vi "ProdaNG.Configurator.vi"() -> ()   [LabVIEW 2016]
uses:
  ProdaNG.Tree.TestViewMode.ctl
  ProdaNG.File.Sequence.ctl
  ProdaNG.Tree.Fglb.Value.ctl
  ProdaNG.File.Step.ctl
  ProdaNG.Configurator.DB.ctl
  ProdaNG.Configurator.Config.ctl
  ProdaNG.Configurator.ResultsTimeSpan.ctl
  Controls/ProdaNG.Product.ctl
  ProdaNG.Configurator.State.ctl
  <vilib>/Utility/error.llb/DialogTypeEnum.ctl
  <vilib>/Utility/miscctls.llb/LVNodeAndColumnTypeDef.ctl
  ProdaNG.Configurator.Glb.vi
panel:
  out "Products":T1[](array[typedef])
  out "DBtime":timestamp
  out "SelectedFile":path
  out "Progress":bool caption="Please wait..."
  out "Hider":bool
  out "PrevTabState":i32
  in  "ButtonResults":bool
  out "SlotInUse":i32
  in  "ButtonTest":bool
  in  "ButtonParts":bool
  out "DB":T2
  out "ProfInfo":string[](array[string])
  in  "TestTreeView":T3
  out "FPref":refnum<vi>
  out "FileContent":T4
  in  "MainTab":enum32{"Parts", "Test", "Results"}(tab)
  in  "ButtonConnect":bool caption="Check"
  out "HiderParts":bool
  in  "ButtonGoToResults":bool
  in  "ButtonGoToTest":bool caption="Accept"
  in  "VariantFilter":string caption="Wabco Part Filter"
  in  "ButtonRefreshTreeProc":bool caption="Refresh"
  in  "ProcTree":string(tree) caption="Found 4 wabco parts"
  out "Identification":T7
  out "Process Found":bool
  in  "color legend 4":u32(colorbox)=16448250 caption="- wabco part"
  in  "color legend 5":u32(colorbox)=12058551 caption="- process"
  in  "color legend 6":u32(colorbox)=16777134 caption="- process step"
  in  "ButtonReloadDB":bool caption="Refresh"
  in  "Configuration":T8={"ShowUnreleased"=TRUE, "Param1"="StepIndex", "ParamStartIdx"=0, "Slots"=1} {"Slots" min=1 max=2; "ParamStartIdx" min=0 max=1}
  in  "TestTree.OpenCloseAll":bool caption="collapse all"
  in  "ButtonSaveToFile":bool
  out "FileInUse":string
  in  "ButtonCloseFile":bool
  in  "ButtonExportFile":bool
  in  "ButtonOpenFile":bool
  in  "color legend 1":u32(colorbox)=16448250 caption="- item synchronized"
  in  "color legend 3":u32(colorbox)=16744576 caption="- item value changed"
  in  "color legend 2":u32(colorbox)=16777147 caption="- new item in file (not found in DB)"
  in  "ButtonUnreleaseAll":bool
  in  "ButtonReleaseAll":bool
  in  "ButtonUnrelease":bool
  in  "ButtonRelease":bool
  in  "ButtonDeleteAll":bool
  in  "ButtonAdd":bool
  in  "ButtonEdit":bool
  in  "ButtonDelete":bool
  in  "TestTree":string[](tree)
  in  "ButtonRefreshTestTree":bool
  in  "ResultsAmount":i32 caption="Span" min=0 max=100
  in  "ResultsSpan":T9
  in  "Results.TimeTo":timestamp caption="Time To" format="%<%x %X>T"
  in  "Results.TimeFrom":timestamp caption="Time From" format="%<%x %X>T"
  in  "ProductList":i32[](listbox) caption="Products #208"
  in  "color legend 9":u32(colorbox)=16448250 caption="- value ok"
  in  "color legend 8":u32(colorbox)=16744576 caption="- value nok"
  in  "color legend 7":u32(colorbox)=13816530 caption="- value missing"
  in  "ResultsTree":string[](tree)
  in  "ButtonRefreshResultTree":bool
  in  "ProductListSelectAll":enum8{"False", "True", "Mixed"}(c332) caption="All"
  in  "Starthere":bool
  out "Status":string
  out "DBStatus":string
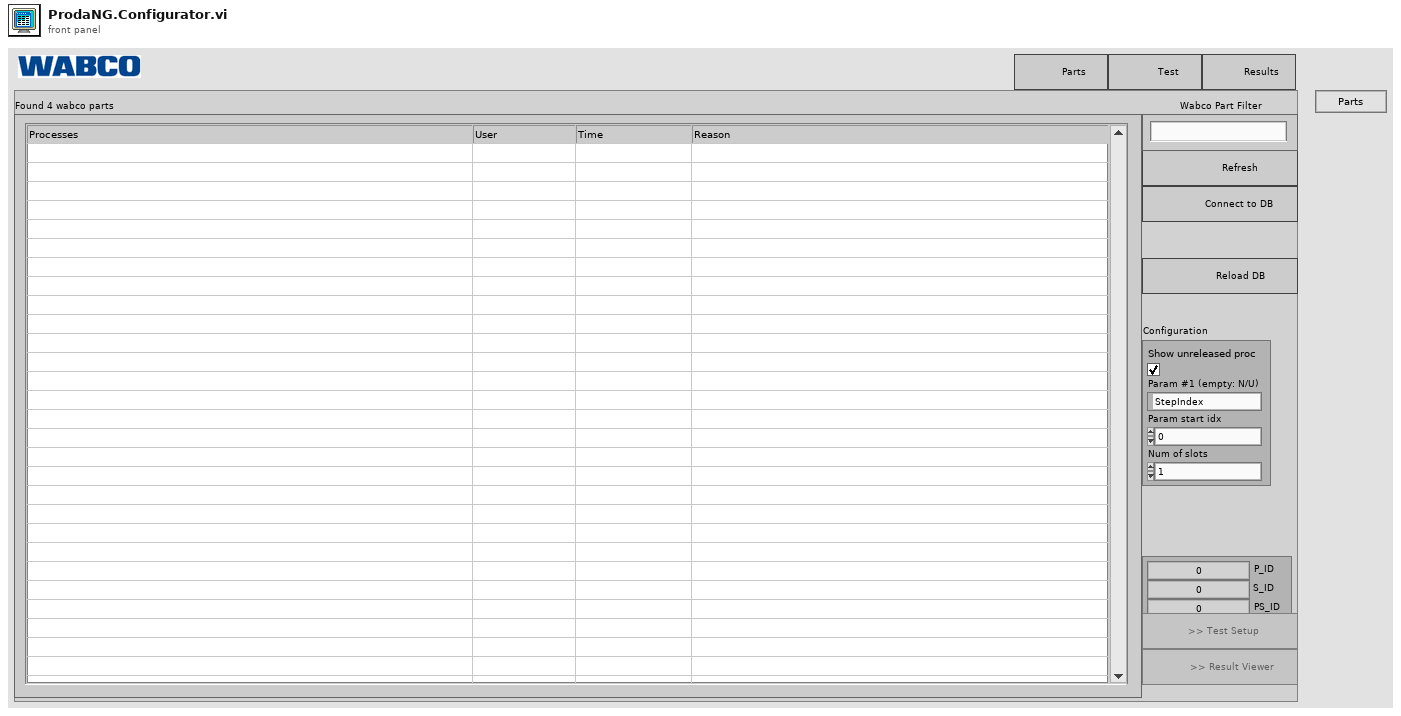
[diagram p1: front panel]
types:
  T1 = typedef "ProdaNG.Product.ctl" = cluster{"c_id":string, "wabcoPartId":i32, "serialNumber":string, "comment":string, "individual":i32, "crProcessStepId":i32, "mdProcessStepId":i32, "crTime":string, "mdTime":string}
  T2 = typedef "ProdaNG.Configurator.DB.ctl" = enum16{"other", "WPL", "WPK"}
  T3 = typedef "ProdaNG.Tree.TestViewMode.ctl" = enum16{"All", "Released", "Unreleased"}
  T4 = typedef "ProdaNG.File.Sequence.ctl" = cluster{"PP":T5[], "TS":T6[]}
  T5 = typedef "ProdaNG.Tree.Fglb.Value.ctl" = cluster{"desc":string, "order":i32, "value1":dbl, "value2":dbl, "unit":i32}
  T6 = typedef "ProdaNG.File.Step.ctl" = cluster{"TS":T5, "TP":T5[], "TV":T5[]}
  T7 = cluster{"P_ID":i32, "S_ID":i32, "PS_ID":i32, "WP_ID":i32}
  T8 = typedef "ProdaNG.Configurator.Config.ctl" = cluster{"ShowUnreleased":bool, "Param1":string, "ParamStartIdx":i32, "Slots":i32}
  T9 = typedef "ProdaNG.Configurator.ResultsTimeSpan.ctl" = enum16{"Custom", "Shift(s)", "Hour(s)", "Day(s)", "Week(s)", "Month(s)"}
  T10 = typedef "ProdaNG.Configurator.State.ctl" = enum16{"Disconnected", "Connected", "ProcessFound"}
  T11 = enum8{"Enabled", "Disabled", "Disabled and Grayed Out"}
  T12 = cluster{"processId":i32, "systemId":i32, "processStepId":i32, "wabcoPartId":i32}
  T13 = typedef "DialogTypeEnum.ctl" = enum16{"no dialog", "OK message", "continue or stop message", "auto error handling dialog", "OK message + warnings", "continue/stop + warnings"}
  T14 = typedef "LVNodeAndColumnTypeDef.ctl" = cluster{"Node":string, "Column":i32}
  T15 = enum16{"Custom", "Shift(s)", "Hour(s)", "Day(s)", "Week(s)", "Month(s)"}
  T16 = typedef "LVPositionTypeDef.ctl" = cluster{"Left":i32, "Top":i32}
  T17 = typedef "ProdaNG.ProdutionLine.ctl" = cluster{"i_id":i32, "description":string}
  T18 = typedef "ProdaNG.System.ctl" = cluster{"i_id":i32, "description":string}
  T19 = typedef "ProdaNG.Process.ctl" = cluster{"i_id":i32, "productionLineId":i32, "releaseId":i32, "contentId":string, "previewId":string, "mdReason":string, "mdUser":string, "mdTime":string, "description":string}
  T20 = typedef "ProdaNG.WabcoPart.ctl" = cluster{"i_id":i32, "workCenterId":i32, "contentId":string, "previewId":string, "mdReason":string, "mdUser":string, "mdTime":string, "productName":string, "wabcoNumber":string}
  T21 = typedef "ProdaNG.ProcessStep.ctl" = cluster{"i_id":i32, "processId":i32, "systemId":i32, "releaseId":i32, "processSequence":i32, "limitYellow":dbl, "limitRed":dbl, "mdReason":string, "mdUser":string, "mdTime":string, "filename":string, "transfer":string, "description":string}
  T22 = typedef "ProdaNG.Tree.Fglb.Data.ctl" = cluster{"tag":string, "row":i32, "element":T23, "idx1":i32, "idx2":i32, "file":bool}
  T23 = typedef "ProdaNG.Tree.Fglb.Element.ctl" = enum16{"-", "PP", "TS", "TP", "TV"}
  T24 = typedef "ProdaNG.UnitSimple.ctl" = cluster{"name":string, "i_id":i32}
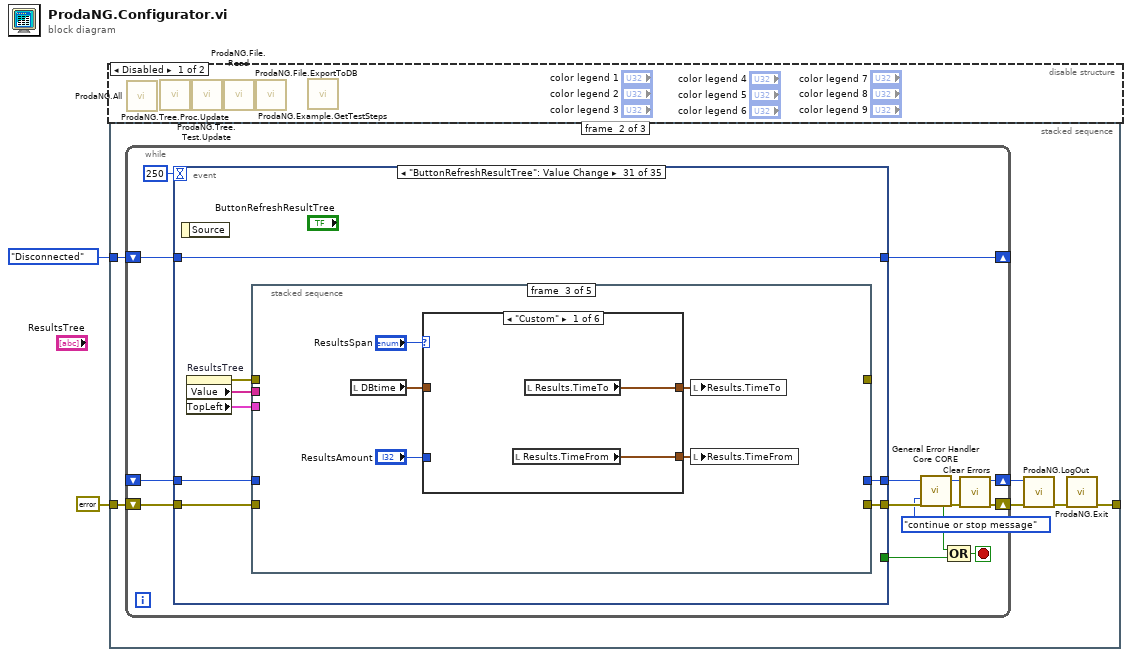
[diagram p0: block diagram]
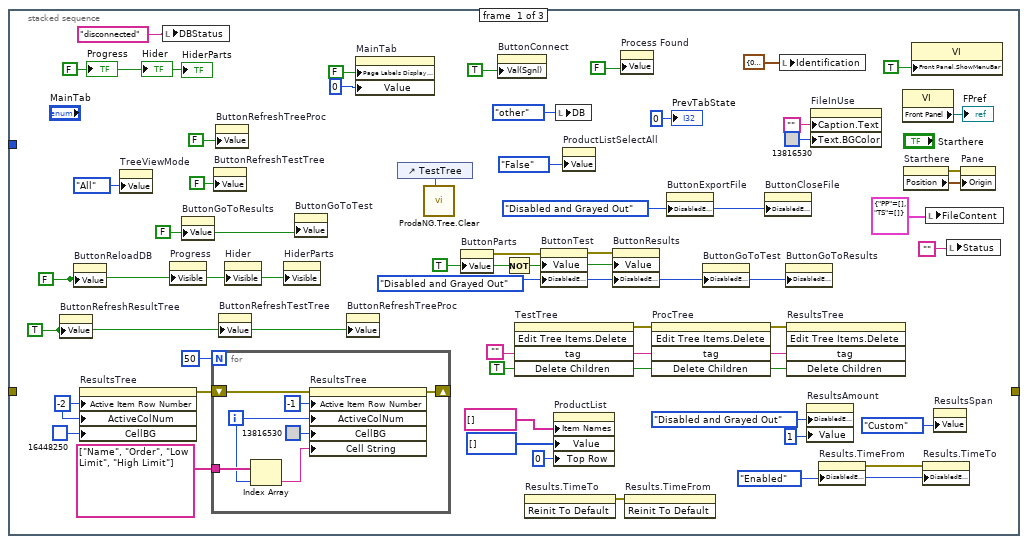
[diagram p2: hidden frame]
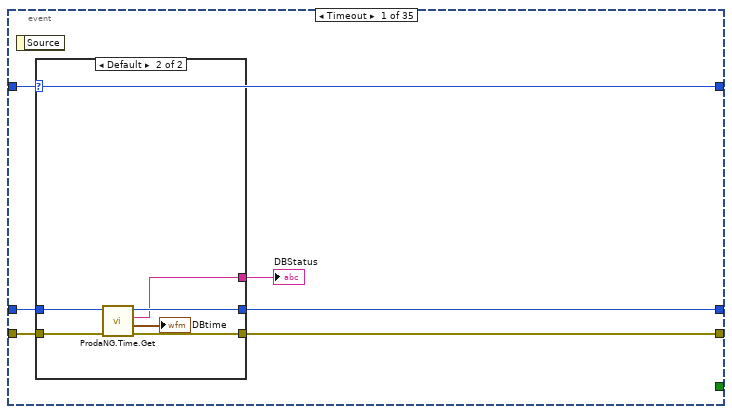
[diagram p3: hidden frame]
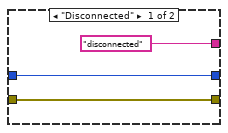
[diagram p4: hidden frame]
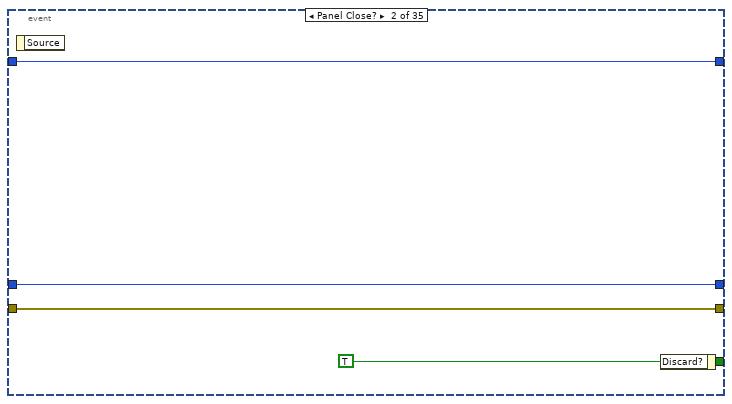
[diagram p5: hidden frame]
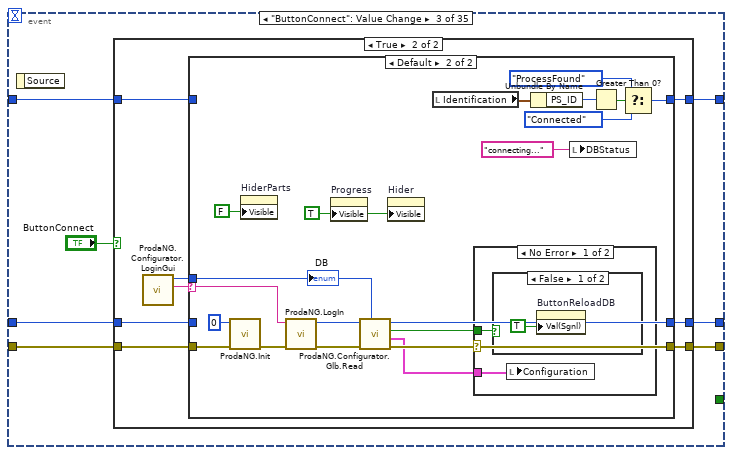
[diagram p6: hidden frame]
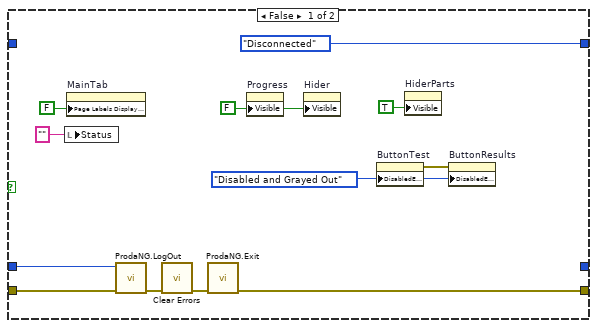
[diagram p7: hidden frame]
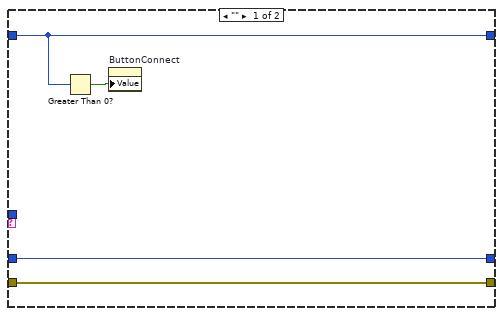
[diagram p8: hidden frame]
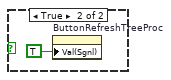
[diagram p9: hidden frame]
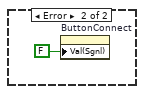
[diagram p10: hidden frame]
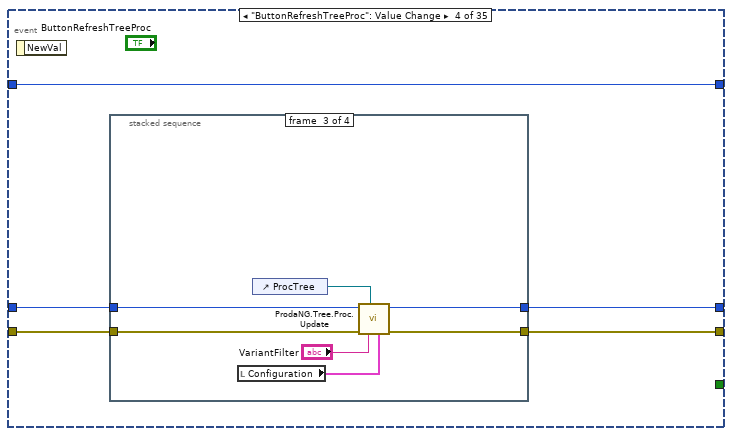
[diagram p11: hidden frame]
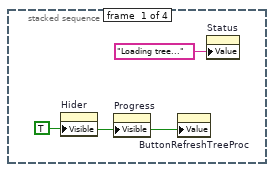
[diagram p12: hidden frame]
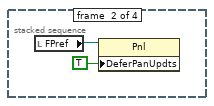
[diagram p13: hidden frame]
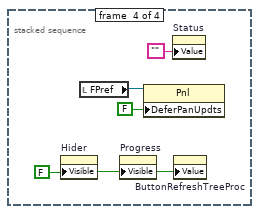
[diagram p14: hidden frame]
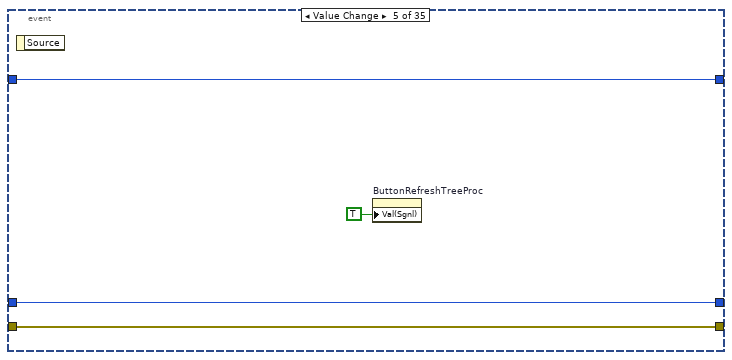
[diagram p15: hidden frame]
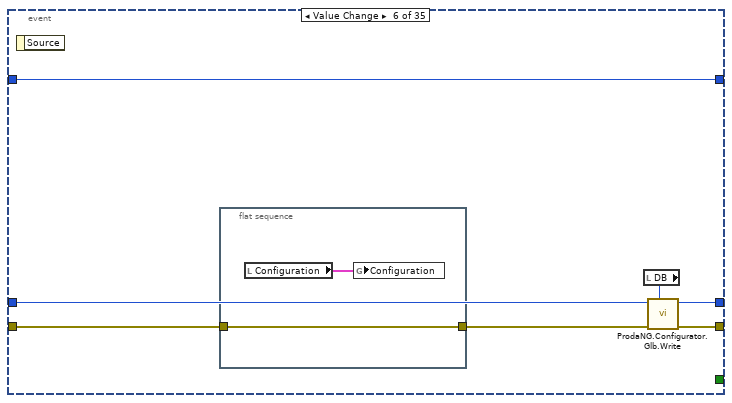
[diagram p16: hidden frame]
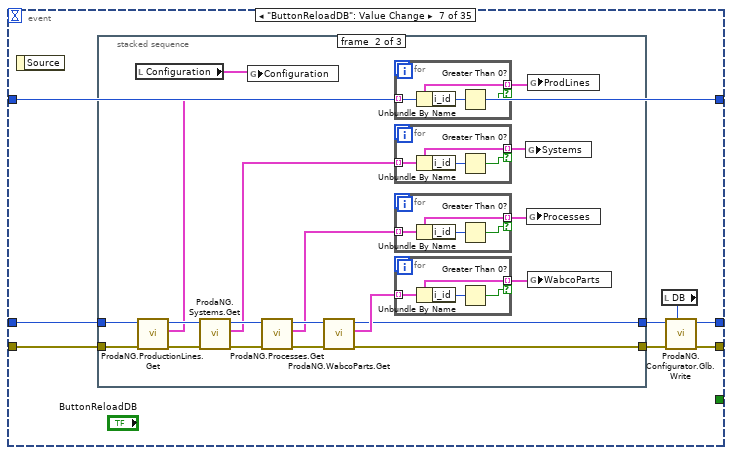
[diagram p17: hidden frame]
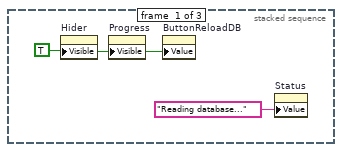
[diagram p18: hidden frame]
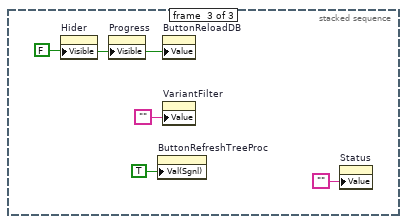
[diagram p19: hidden frame]
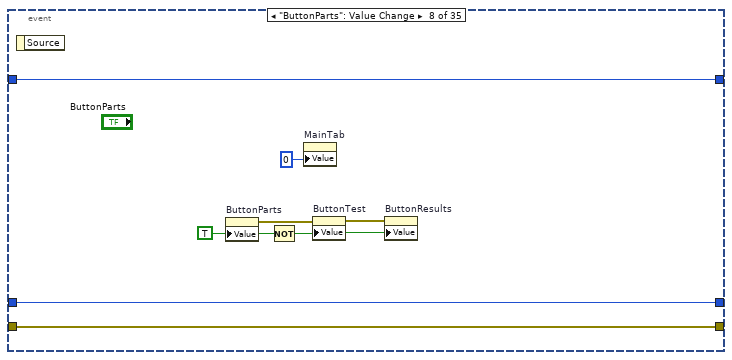
[diagram p20: hidden frame]
diagram:
  n1 = disable-structure shown="Disabled" {
    frame Disabled {
      n2 = call "ProdaNG.All.vi"() -> ()  [unwired: 1 in]
      n3 = call "ProdaNG.Tree.Proc.Update.vi"() -> ()  [unwired: 10 in, 2 out]
      n4 = call "ProdaNG.Tree.Test.Update.vi"() -> ()  [unwired: 8 in, 4 out]
      n5 = call "ProdaNG.File.Read.vi"() -> ()  [unwired: 9 in, 3 out]
      n6 = call "ProdaNG.File.ExportToDB.vi"() -> ()  [unwired: 10 in, 2 out]
      n7 = call "ProdaNG.Example.GetTestSteps.vi"() -> ()  [unwired: 12 in]
    }
    frame Enabled {
    }
  }
  n8 = stacked-sequence {
    tunnel: ProdaNG.Configurator.State."Disconnected" ("State") -> [_ w62 _]
    tunnel: [_ w60 _] -> _
    tunnel: errorcluster {"status"=FALSE, "code"=0, "source"=""} ("error out") -> [_ w59 _]
    frame #0 {
      w5 = T11."Enabled" ("Disabled")
      w11 = TRUE ("Value (Signaling)")
      w17 = -2 ("Active Item:Row Number")
      w23 = TRUE ("Delete Children?")
      w24 = ""
      w28 = FALSE ("Progress")
      w29 = FALSE ("ButtonGoToResults")
      w31 = T11."Disabled and Grayed Out" ("Disabled")
      w36 = TRUE ("ButtonPartList")
      w27 = FALSE ("Visible")
      w45 = T11."Disabled and Grayed Out" ("Disabled")
      n9 = property on="ButtonRefreshResultTree" class="Bool (strict)"("Value"=w11) -> ()  [unwired: 2 in, 2 out]
      n10 = property on="ButtonReloadDB" class="Bool (strict)"("Value"=w27) -> ()  [unwired: 2 in, 2 out]
      n11 = property on="ResultsTree" class="Tree (strict)"("Active Item Row Number"=w17, "ActiveColNum"=w17, "CellBG"=u32 16448250) -> (error out=w18:errorcluster)  [unwired: 2 in, 1 out]
      n12 = property on="TreeViewMode" class="Enum (strict)"("Value"=ProdaNG.Tree.TestViewMode."All" ("TreeViewMode")) -> ()  [unwired: 2 in, 2 out]
      n13 = local write "DBStatus"("disconnected" ("string")) -> ()
      n14 = property on="Progress" class="Bool (strict)"("Visible"=w27) -> ()  [unwired: 2 in, 2 out]
      n15 = property on="ButtonGoToResults" class="Bool (strict)"("Value"=w29) -> ()  [unwired: 2 in, 2 out]
      n16 = for {
        N: 50 -> [_]
        tunnel: string[] ["Name", "Order", "Low Limit", "High Limit"] -> [w55]
        shift-right: [w53] -> _
        shift-left: w18 -> [w58]
        i -> [w52]
        n17 = Index Array(array=w55, index=w52) -> (element=w54:string)
        n18 = property on="ResultsTree" class="Tree (strict)"(error in=w58, "Active Item Row Number"=-1 ("Active Item:Row Number"), "ActiveColNum"=w52, "CellBG"=u32 13816530, "Cell String"=w54) -> (error out=w53:errorcluster)  [unwired: 1 in, 1 out]
      }
      n19 = property on="ButtonRefreshTestTree" class="Bool (strict)"("Value"=FALSE ("ButtonRefreshSystem")) -> ()  [unwired: 2 in, 2 out]
      n20 = property on="ButtonRefreshTreeProc" class="Bool (strict)"("Value"=FALSE ("Value (Signaling)")) -> ()  [unwired: 2 in, 2 out]
      n21 = property on="ButtonRefreshTestTree" class="Bool (strict)"("Value"=w11) -> ()  [unwired: 2 in, 2 out]
      n22 = property on="Hider" class="Bool (strict)"("Visible"=w27) -> ()  [unwired: 2 in, 2 out]
      n23 = property on="HiderParts" class="Bool (strict)"("Visible"=w27) -> ()  [unwired: 2 in, 2 out]
      n24 = property on="ButtonGoToTest" class="Bool (strict)"("Value"=w29) -> ()  [unwired: 2 in, 2 out]
      n25 = property on="ButtonRefreshTreeProc" class="Bool (strict)"("Value"=w11) -> ()  [unwired: 2 in, 2 out]
      n26 = property on="MainTab" class="TabCtl (strict)"("Page Labels Display Visible?"=FALSE, "Value"=0) -> ()  [unwired: 2 in, 2 out]
      n27 = control-ref of="TestTree"() -> (w49:refnum<vi>)
      n28 = call "ProdaNG.Tree.Clear.vi"("TestStepsTree"=w49) -> ()  [unwired: 10 in, 1 out]
      n29 = property on="ButtonParts" class="Bool (strict)"("Value"=w36) -> (error out=w35:errorcluster)  [unwired: 2 in, 1 out]
      n30 = property on="ButtonConnect" class="Bool (strict)"("Val(Sgnl)"=TRUE ("ButtonConnect")) -> ()  [unwired: 2 in, 2 out]
      n31 = Not(x=w36) -> (.not. x?=w33:bool)
      n32 = invoke on="TestTree" class="Tree (strict)" method="Edit Tree Items.Delete"("tag"=w24, "Delete Children"=w23) -> (error out=w26:errorcluster)  [unwired: 3 in, 4 out]
      n33 = invoke on="Results.TimeTo" class="AbsTime (strict)" method="Reinit To Default"() -> (error out=w3:errorcluster)  [unwired: 3 in, 2 out]
      n34 = property on="ButtonTest" class="Bool (strict)"(error in=w35, "Value"=w33, "DisabledEnum"=w31) -> (error out=w34:errorcluster)  [unwired: 1 in, 1 out]
      n35 = property on="ProductList" class="LstBox (strict)"("Item Names"=string[] [], "Value"=i32[] [] ("ProductList"), "Top Row"=0) -> ()  [unwired: 2 in, 2 out]
      n36 = local write "DB"(ProdaNG.Configurator.DB."other" ("DB")) -> ()
      n37 = property on="ProductListSelectAll" class="MixedCheckbox (strict)"("Value"=enum8{"False", "True", "Mixed"}."False" ("Mixed Checkbox")) -> ()  [unwired: 2 in, 2 out]
      n38 = property on="ButtonResults" class="Bool (strict)"(error in=w34, "Value"=w33, "DisabledEnum"=w31) -> ()  [unwired: 1 in, 2 out]
      n39 = property on="Process Found" class="Bool (strict)"("Value"=FALSE ("Visible")) -> ()  [unwired: 2 in, 2 out]
      n40 = invoke on="Results.TimeFrom" class="AbsTime (strict)" method="Reinit To Default"(error in=w3) -> ()  [unwired: 2 in, 3 out]
      n41 = invoke on="ProcTree" class="Tree (strict)" method="Edit Tree Items.Delete"(error in=w26, "tag"=w24, "Delete Children"=w23) -> (error out=w25:errorcluster)  [unwired: 2 in, 4 out]
      n42 = property on="ButtonExportFile" class="Bool (strict)"("DisabledEnum"=w45) -> ()  [unwired: 2 in, 2 out]
      n43 = property on="ButtonGoToTest" class="Bool (strict)"("DisabledEnum"=w31) -> ()  [unwired: 2 in, 2 out]
      n44 = property on="ButtonCloseFile" class="Bool"("DisabledEnum"=w45) -> ()  [unwired: 2 in, 2 out]
      n45 = local write "Identification"(T12 {"processId"=0, "systemId"=0, "processStepId"=0, "wabcoPartId"=0} ("Identification")) -> ()
      n46 = property on="ButtonGoToResults" class="Bool (strict)"("DisabledEnum"=w31) -> ()  [unwired: 2 in, 2 out]
      n47 = invoke on="ResultsTree" class="Tree (strict)" method="Edit Tree Items.Delete"(error in=w25, "tag"=w24, "Delete Children"=w23) -> ()  [unwired: 2 in, 5 out]
      n48 = property on="ResultsAmount" class="DigNum (strict)"("DisabledEnum"=T11."Disabled and Grayed Out" ("Disabled"), "Value"=1 ("ResultsAmount")) -> ()  [unwired: 2 in, 2 out]
      n49 = property on="FileInUse" class="Str"("Caption.Text"="", "Text.BGColor"=u32 13816530) -> ()  [unwired: 2 in, 2 out]
      n50 = property on="Results.TimeFrom" class="AbsTime (strict)"("DisabledEnum"=w5) -> (error out=w6:errorcluster)  [unwired: 2 in, 1 out]
      n51 = property class="VI"() -> ("Front Panel"=→"FPref":refnum<vi>)  [unwired: 2 in, 2 out]
      n52 = property on="Starthere" class="Bool (strict)"() -> (error out=w10:errorcluster, "Position"=w9:T16)  [unwired: 2 in, 1 out]
      n53 = property class="VI"("Front Panel.ShowMenuBar"=TRUE ("Front Panel Window:Show Menu Bar")) -> ()  [unwired: 2 in, 2 out]
      n54 = property on="Results.TimeTo" class="AbsTime (strict)"(error in=w6, "DisabledEnum"=w5) -> ()  [unwired: 1 in, 2 out]
      n55 = local write "FileContent"(T4 {"PP"=[], "TS"=[]} ("Seq")) -> ()
      n56 = property on="ResultsSpan" class="Enum (strict)"("Value"=ProdaNG.Configurator.ResultsTimeSpan."Custom" ("ResultsSpan")) -> ()  [unwired: 2 in, 2 out]
      n57 = local write "Status"("") -> ()
      n58 = property on="Pane" class="Pane"(error in=w10, "Origin"=w9) -> ()  [unwired: 1 in, 2 out]
      "PrevTabState" <- 0 ("PrevTabState")
      "Hider" <- w28
      "Progress" <- w28
      "HiderParts" <- w28
    }
    frame #1 {
      n59 = while {
        shift-right: [w72] -> w63
        shift-left: w59 -> [w76]
        shift-right: [w77] -> w64
        shift-left: _ -> [w75]
        shift-right: [w65] -> _
        shift-left: w62 -> [w73]
        stop <- w68 stop-if-true
        n60 = event shown="[30] \"ButtonRefreshResultTree\": Value Change" {
          selector: _ -> [_ _ _ _ _ _ _ _ _ _ _ _ _ _ _ _ _ _ _ _ _ _ _ _ _ _ _ _ _ _ _ _ _ _ _]
          dyn-events: _ -> [_ _ _ _ _ _ _ _ _ _ _ _ _ _ _ _ _ _ _ _ _ _ _ _ _ _ _ _ _ _ _ _ _ _ _]
          timeout: 250 -> [_ _ _ _ _ _ _ _ _ _ _ _ _ _ _ _ _ _ _ _ _ _ _ _ _ _ _ _ _ _ _ _ _ _ _]
          tunnel: [w81 w93 w102 w154 w173 w178 w187 w232 w241 w249 w264 w273 w291 w348 w360 w370 w430 w454 w464 w508 w552 w596 w644 w680 w723 w760 w799 w848 w856 w886 w931 w1018 w1027 w1029 w1042] -> w77
          tunnel: w76 -> [w83 w94 w103 w153 w174 w177 w189 w233 w242 w250 w265 w274 w294 w349 w361 w364 w444 w455 w463 w507 w551 w595 w638 w677 w726 w763 w802 w849 w857 w887 w925 w1017 w1026 w1030 w1044]
          tunnel: w75 -> [w82 w93 w99 w155 w173 w178 w188 w232 w241 w249 w264 w273 w293 w348 w360 w368 w430 w454 w466 w510 w554 w598 w637 w674 w725 w762 w799 w848 w858 w888 w929 w1018 w1027 w1029 w1043]
          tunnel: [w78 w94 w101 w152 w174 w179 w185 w233 w242 w250 w265 w274 w292 w349 w361 w363 w428 w455 w465 w509 w553 w597 w645 w681 w724 w761 w801 w849 w855 w899 w924 w1017 w1026 w1030 w1041] -> w71
          tunnel: [w80 w96 w98 w156 w175 w181 w190 w235 w243 w251 w266 w282 w295 ProdaNG.Configurator.State."ProcessFound" ("State") ProdaNG.Configurator.State."ProcessFound" ("State") w369 w445 w456 w457 w501 w545 w589 w643 w679 w722 w759 w805 w852 w859 w900 w930 w1019 w1028 w1034 w1045] -> w65
          tunnel: w73 -> [w80 w96 w97 w156 w175 w181 w190 w235 w243 w251 w266 w282 w295 _ _ w369 w445 w456 w457 w501 w545 w589 w643 w679 w722 w759 w805 w852 w859 w900 w930 w1019 w1028 w1034 w1045]
          tunnel: [_ w95 _ _ _ _ _ _ _ _ _ _ _ _ _ _ _ _ _ _ _ _ _ _ _ _ _ _ _ _ _ _ _ _ _] -> w69
          event Timeout {
            n61 = event-data() -> ()  [unwired: 1 in, 1 out]
            n62 = case shown="Default" w80 {
              tunnel: w83 -> [w86 w92]
              tunnel: [w86 w91] -> w78
              tunnel: w82 -> [w85 w90]
              tunnel: [w85 w89] -> w81
              tunnel: ["disconnected" ("string") w88] -> w79
              frame "Disconnected" {
              }
              frame Default {
                n63 = call "ProdaNG.Time.Get.vi"("error in"=w92, "dbHandleIn"=w90) -> ("error out"=w91:errorcluster, "time"=→"DBtime":timestamp, "timeStr"=w88:string, "dbHandle"=w89:i32)  [unwired: 5 in]
              }
            }
            "DBStatus" <- w79
          }
          event Panel Close? {
            w95 = TRUE ("Discard?")
            n64 = event-data() -> ()  [unwired: 1 in, 1 out]
            n65 = event-data("Discard?"=w95) -> ()  [unwired: 1 in, 1 out]
          }
          event "ButtonConnect": Value Change {
            n66 = event-data() -> ()  [unwired: 1 in, 1 out]
            n67 = case shown="True" "ButtonConnect" {
              tunnel: w103 -> [w114 w123]
              tunnel: [_ w121] -> w102
              tunnel: [w113 w122] -> w101
              tunnel: w99 -> [w112 w119]
              tunnel: [ProdaNG.Configurator.State."Disconnected" ("State") w117] -> w98
              tunnel: w97 -> [_ w118]
              frame False {
                w104 = FALSE ("Visible")
                w106 = T11."Disabled and Grayed Out" ("Disabled")
                n68 = local write "Status"("" ("Status")) -> ()
                n69 = property on="MainTab" class="TabCtl (strict)"("Page Labels Display Visible?"=FALSE) -> ()  [unwired: 2 in, 2 out]
                n70 = call "ProdaNG.LogOut.vi"("error in"=w114, "dbHandleIn"=w112) -> ("error out"=w115:errorcluster)  [unwired: 9 in]
                n71 = call <vilib>:"Clear Errors.vi"("error in (no error)"=w115) -> ("error out"=w107:errorcluster)  [unwired: 5 in, 1 out]
                n72 = call "ProdaNG.Exit.vi"("error in (no error)"=w107) -> ("error out"=w113:errorcluster)  [unwired: 10 in]
                n73 = property on="Progress" class="Bool (strict)"("Visible"=w104) -> ()  [unwired: 2 in, 2 out]
                n74 = property on="Hider" class="Bool (strict)"("Visible"=w104) -> ()  [unwired: 2 in, 2 out]
                n75 = property on="ButtonTest" class="Bool (strict)"("DisabledEnum"=w106) -> (error out=w105:errorcluster)  [unwired: 2 in, 1 out]
                n76 = property on="HiderParts" class="Bool (strict)"("Visible"=TRUE) -> ()  [unwired: 2 in, 2 out]
                n77 = property on="ButtonResults" class="Bool (strict)"(error in=w105, "DisabledEnum"=w106) -> ()  [unwired: 1 in, 2 out]
              }
              frame True {
                n78 = call "ProdaNG.Configurator.LoginGui.vi"() -> ("ConnectionString"=w120:string, "DB"=w116:T2)  [unwired: 10 in]
                n79 = case shown="Default" w120 {
                  selector: w120 -> [_ w143]
                  tunnel: w123 -> [w126 w144]
                  tunnel: [w126 w135] -> w122
                  tunnel: [w127 w129] -> w121
                  tunnel: w119 -> [w127 _]
                  tunnel: w118 -> [w125 _]
                  tunnel: [w125 w137] -> w117
                  tunnel: w116 -> [_ w136]
                  frame "" {
                    n80 = Greater Than 0?(x=w125) -> (x > 0?=w124:bool)
                    n81 = property on="ButtonConnect" class="Bool (strict)"("Value"=w124) -> ()  [unwired: 2 in, 2 out]
                  }
                  frame Default {
                    w132 = TRUE ("Visible")
                    n82 = call "ProdaNG.Init.vi"("error in (no error)"=w144, "numContexts (0: unlimited)"=0 ("numContexts")) -> ("error out"=w145:errorcluster)  [unwired: 9 in]
                    n83 = property on="HiderParts" class="Bool (strict)"("Visible"=FALSE) -> ()  [unwired: 2 in, 2 out]
                    n84 = call "ProdaNG.LogIn.vi"("error in"=w145, "ConnectionString"=w143) -> ("error out"=w130:errorcluster, "dbHandle"=w129:i32)  [unwired: 7 in, 1 out]
                    n85 = property on="Progress" class="Bool (strict)"("Visible"=w132) -> ()  [unwired: 2 in, 2 out]
                    n86 = call "ProdaNG.Configurator.Glb.Read.vi"("DB"=w136, "error in (no error)"=w130) -> ("error out"=w135:errorcluster, "Configuration"=w128:T8, "Data found"=w134:bool)  [unwired: 7 in]
                    n87 = property on="Hider" class="Bool (strict)"("Visible"=w132) -> ()  [unwired: 2 in, 2 out]
                    n88 = local read "Identification"() -> (w138:T7)
                    n89 = case shown="No Error" w135 {
                      tunnel: w134 -> [w148 _]
                      tunnel: w128 -> [w147 _]
                      frame No Error {
                        n90 = case shown="False" w148 {
                          frame False {
                            n91 = property on="ButtonReloadDB" class="Bool (strict)"("Val(Sgnl)"=TRUE ("Value (Signaling)")) -> ()  [unwired: 2 in, 2 out]
                          }
                          frame True {
                            n92 = property on="ButtonRefreshTreeProc" class="Bool (strict)"("Val(Sgnl)"=TRUE ("Value (Signaling)")) -> ()  [unwired: 2 in, 2 out]
                          }
                        }
                        n93 = local write "Configuration"(w147) -> ()
                      }
                      frame Error {
                        n94 = property on="ButtonConnect" class="Bool (strict)"("Val(Sgnl)"=FALSE ("Value (Signaling)")) -> ()  [unwired: 2 in, 2 out]
                      }
                    }
                    n95 = Unbundle By Name(w138) -> ("PS_ID"=w139:i32)
                    n96 = local write "DBStatus"("connecting..." ("Front Panel Window:Title")) -> ()
                    n97 = Greater Than 0?(x=w139) -> (x > 0?=w140:bool)
                    n98 = Select(t=ProdaNG.Configurator.State."ProcessFound" ("State"), s=w140, f=ProdaNG.Configurator.State."Connected" ("State")) -> (s? t:f=w137:T10)
                    "DB" <- w136
                  }
                }
              }
            }
          }
          event "ButtonRefreshTreeProc": Value Change {
            n99 = event-data() -> ()  [unwired: 1 in, 1 out]
            n100 = stacked-sequence {
              tunnel: w155 -> [_ _ w167 _]
              tunnel: [_ _ w166 _] -> w154
              tunnel: w153 -> [_ _ w163 _]
              tunnel: [_ _ w162 _] -> w152
              frame #0 {
                w157 = TRUE ("Visible")
                n101 = property on="Hider" class="Bool (strict)"("Visible"=w157) -> ()  [unwired: 2 in, 2 out]
                n102 = property on="Progress" class="Bool (strict)"("Visible"=w157) -> ()  [unwired: 2 in, 2 out]
                n103 = property on="ButtonRefreshTreeProc" class="Bool (strict)"("Value"=w157) -> ()  [unwired: 2 in, 2 out]
                n104 = property on="Status" class="Str"("Value"="Loading tree..." ("Status")) -> ()  [unwired: 2 in, 2 out]
              }
              frame #1 {
                n105 = local read "FPref"() -> (w159:refnum<vi>)
                n106 = property class="Pnl"(reference=w159, "DeferPanUpdts"=TRUE ("Defer Panel Updates")) -> ()  [unwired: 1 in, 2 out]
              }
              frame #2 {
                n107 = local read "Configuration"() -> (w161:T8)
                n108 = control-ref of="ProcTree"() -> (w165:refnum<vi>)
                n109 = call "ProdaNG.Tree.Proc.Update.vi"("Configuration"=w161, "VariantFilter"="VariantFilter", "Tree"=w165, "error in (no error)"=w163, "dbHandle in"=w167) -> ("error out"=w162:errorcluster, "dbHandle out"=w166:i32)  [unwired: 5 in]
              }
              frame #3 {
                w168 = FALSE ("Visible")
                n110 = property on="Hider" class="Bool (strict)"("Visible"=w168) -> ()  [unwired: 2 in, 2 out]
                n111 = local read "FPref"() -> (w170:refnum<vi>)
                n112 = property on="Progress" class="Bool (strict)"("Visible"=w168) -> ()  [unwired: 2 in, 2 out]
                n113 = property class="Pnl"(reference=w170, "DeferPanUpdts"=FALSE ("Defer Panel Updates")) -> ()  [unwired: 1 in, 2 out]
                n114 = property on="Status" class="Str"("Value"="") -> ()  [unwired: 2 in, 2 out]
                n115 = property on="ButtonRefreshTreeProc" class="Bool (strict)"("Value"=w168) -> ()  [unwired: 2 in, 2 out]
              }
            }
          }
          event Value Change {
            n116 = event-data() -> ()  [unwired: 1 in, 1 out]
            n117 = property on="ButtonRefreshTreeProc" class="Bool (strict)"("Val(Sgnl)"=TRUE ("Value (Signaling)")) -> ()  [unwired: 2 in, 2 out]
          }
          event Value Change {
            n118 = event-data() -> ()  [unwired: 1 in, 1 out]
            n119 = flat-sequence {
              tunnel: w177 -> [w182]
              tunnel: [w182] -> w176
              frame #0 {
                n120 = local read "Configuration"() -> (w183:T8)
                n121 = global write "ProdaNG.Configurator.Glb.vi" "Configuration"(w183) -> ()
              }
            }
            n122 = local read "DB"() -> (w180:T2)
            n123 = call "ProdaNG.Configurator.Glb.Write.vi"("DB"=w180, "error in (no error)"=w176) -> ("error out"=w179:errorcluster)  [unwired: 9 in]
          }
          event "ButtonReloadDB": Value Change {
            n124 = event-data() -> ()  [unwired: 1 in, 1 out]
            n125 = stacked-sequence {
              tunnel: w189 -> [_ w202 _]
              tunnel: w188 -> [_ w208 _]
              tunnel: [_ w207 _] -> w187
              tunnel: [_ w206 _] -> w186
              frame #0 {
                w191 = TRUE ("Visible")
                n126 = property on="Hider" class="Bool (strict)"("Visible"=w191) -> ()  [unwired: 2 in, 2 out]
                n127 = property on="Progress" class="Bool (strict)"("Visible"=w191) -> ()  [unwired: 2 in, 2 out]
                n128 = property on="ButtonReloadDB" class="Bool (strict)"("Value"=w191) -> ()  [unwired: 2 in, 2 out]
                n129 = property on="Status" class="Str"("Value"="Reading database..." ("Status")) -> ()  [unwired: 2 in, 2 out]
              }
              frame #1 {
                n130 = local read "Configuration"() -> (w193:T8)
                n131 = call "ProdaNG.ProductionLines.Get.vi"("error in (no error)"=w202, "dbHandleIn"=w208) -> ("error out"=w201:errorcluster, "ProdLines"=w200:T17[], "dbHandle"=w203:i32)  [unwired: 7 in]
                n132 = call "ProdaNG.Systems.Get.vi"("error in (no error)"=w201, "dbHandleIn"=w203) -> ("error out"=w197:errorcluster, "Systems"=w209:T18[], "dbHandle"=w210:i32)  [unwired: 7 in]
                n133 = global write "ProdaNG.Configurator.Glb.vi" "Configuration"(w193) -> ()
                n134 = call "ProdaNG.Processes.Get.vi"("error in (no error)"=w197, "dbHandleIn"=w210) -> ("error out"=w196:errorcluster, "Processes"=w194:T19[], "dbHandle"=w198:i32)  [unwired: 7 in]
                n135 = call "ProdaNG.WabcoParts.Get.vi"("error in (no error)"=w196, "dbHandleIn"=w198) -> ("error out"=w206:errorcluster, "WabcoParts"=w211:T20[], "dbHandle"=w207:i32)  [unwired: 7 in]
                n136 = for {
                  tunnel: w200 -> [w217] mode=indexing
                  tunnel: [w217] -> w199 mode=indexing if=w215
                  n137 = Unbundle By Name(w217) -> ("i_id"=w216:i32)
                  n138 = Greater Than 0?(x=w216) -> (x > 0?=w215:bool)
                }
                n139 = for {
                  tunnel: w209 -> [w223] mode=indexing
                  tunnel: [w223] -> w204 mode=indexing if=w221
                  n140 = Unbundle By Name(w223) -> ("i_id"=w222:i32)
                  n141 = Greater Than 0?(x=w222) -> (x > 0?=w221:bool)
                }
                n142 = for {
                  tunnel: w194 -> [w214] mode=indexing
                  tunnel: [w214] -> w195 mode=indexing if=w212
                  n143 = Unbundle By Name(w214) -> ("i_id"=w213:i32)
                  n144 = Greater Than 0?(x=w213) -> (x > 0?=w212:bool)
                }
                n145 = for {
                  tunnel: w211 -> [w220] mode=indexing
                  tunnel: [w220] -> w205 mode=indexing if=w218
                  n146 = Unbundle By Name(w220) -> ("i_id"=w219:i32)
                  n147 = Greater Than 0?(x=w219) -> (x > 0?=w218:bool)
                }
                n148 = global write "ProdaNG.Configurator.Glb.vi" "Systems"(w204) -> ()
                n149 = global write "ProdaNG.Configurator.Glb.vi" "Processes"(w195) -> ()
                n150 = global write "ProdaNG.Configurator.Glb.vi" "ProdLines"(w199) -> ()
                n151 = global write "ProdaNG.Configurator.Glb.vi" "WabcoParts"(w205) -> ()
              }
              frame #2 {
                w224 = FALSE ("Visible")
                n152 = property on="Hider" class="Bool (strict)"("Visible"=w224) -> ()  [unwired: 2 in, 2 out]
                n153 = property on="Progress" class="Bool (strict)"("Visible"=w224) -> ()  [unwired: 2 in, 2 out]
                n154 = property on="ButtonRefreshTreeProc" class="Bool (strict)"("Val(Sgnl)"=TRUE ("Value (Signaling)")) -> ()  [unwired: 2 in, 2 out]
                n155 = property on="ButtonReloadDB" class="Bool (strict)"("Value"=w224) -> ()  [unwired: 2 in, 2 out]
                n156 = property on="VariantFilter" class="Str"("Value"="") -> ()  [unwired: 2 in, 2 out]
                n157 = property on="Status" class="Str"("Value"="") -> ()  [unwired: 2 in, 2 out]
              }
            }
            n158 = local read "DB"() -> (w184:T2)
            n159 = call "ProdaNG.Configurator.Glb.Write.vi"("DB"=w184, "error in (no error)"=w186) -> ("error out"=w185:errorcluster)  [unwired: 9 in]
          }
          event "ButtonParts": Value Change {
            w231 = TRUE ("ButtonPartList")
            n160 = event-data() -> ()  [unwired: 1 in, 1 out]
            n161 = property on="ButtonParts" class="Bool (strict)"("Value"=w231) -> (error out=w230:errorcluster)  [unwired: 2 in, 1 out]
            n162 = Not(x=w231) -> (.not. x?=w228:bool)
            n163 = property on="MainTab" class="TabCtl (strict)"("Value"=0) -> ()  [unwired: 2 in, 2 out]
            n164 = property on="ButtonTest" class="Bool (strict)"(error in=w230, "Value"=w228) -> (error out=w229:errorcluster)  [unwired: 1 in, 1 out]
            n165 = property on="ButtonResults" class="Bool (strict)"(error in=w229, "Value"=w228) -> ()  [unwired: 1 in, 2 out]
          }
          event "ButtonTest": Value Change {
            w240 = TRUE ("ButtonPartList")
            w236 = 1
            n166 = event-data() -> ()  [unwired: 1 in, 1 out]
            n167 = property on="ButtonTest" class="Bool (strict)"("Value"=w240) -> (error out=w239:errorcluster)  [unwired: 2 in, 1 out]
            n168 = Not(x=w240) -> (.not. x?=w237:bool)
            n169 = property on="ButtonParts" class="Bool (strict)"(error in=w239, "Value"=w237) -> (error out=w238:errorcluster)  [unwired: 1 in, 1 out]
            n170 = property on="MainTab" class="TabCtl (strict)"("Value"=w236) -> ()  [unwired: 2 in, 2 out]
            n171 = property on="ButtonResults" class="Bool (strict)"(error in=w238, "Value"=w237) -> ()  [unwired: 1 in, 2 out]
            n172 = local write "PrevTabState"(w236) -> ()
          }
          event "ButtonResults": Value Change {
            w248 = TRUE ("ButtonPartList")
            w244 = 2
            n173 = event-data() -> ()  [unwired: 1 in, 1 out]
            n174 = property on="ButtonResults" class="Bool (strict)"("Value"=w248) -> (error out=w247:errorcluster)  [unwired: 2 in, 1 out]
            n175 = Not(x=w248) -> (.not. x?=w245:bool)
            n176 = property on="ButtonParts" class="Bool (strict)"(error in=w247, "Value"=w245) -> (error out=w246:errorcluster)  [unwired: 1 in, 1 out]
            n177 = property on="MainTab" class="TabCtl (strict)"("Value"=w244) -> ()  [unwired: 2 in, 2 out]
            n178 = property on="ButtonTest" class="Bool (strict)"(error in=w246, "Value"=w245) -> ()  [unwired: 1 in, 2 out]
            n179 = local write "PrevTabState"(w244) -> ()
          }
          event "ProcTree": Value Change {
            n180 = event-data() -> ("CtlRef"=w261:refnum<vi>, "NewVal"=w257:string)  [unwired: 1 in]
            n181 = call "ProdaNG.Tree.Proc.GetTag.vi"("Tree"=w261, "Tag"=w257) -> ("Process Found"=w258:bool, "Identification"=→"Identification":T7, "ProfInfo"=→"ProfInfo":string[], "SlotNo"=→"SlotInUse":i32)  [unwired: 5 in, 1 out]
            "Process Found" <- w258
            n182 = Select(t=T11."Enabled" ("Disabled"), s=w258, f=T11."Disabled and Grayed Out" ("Disabled")) -> (s? t:f=w253:T11)
            n183 = property on="ButtonTest" class="Bool (strict)"("DisabledEnum"=w253) -> (error out=w255:errorcluster)  [unwired: 2 in, 1 out]
            n184 = property on="ButtonResults" class="Bool (strict)"(error in=w255, "DisabledEnum"=w253) -> (error out=w252:errorcluster)  [unwired: 1 in, 1 out]
            n185 = property on="ButtonGoToTest" class="Bool (strict)"(error in=w252, "DisabledEnum"=w253) -> (error out=w254:errorcluster)  [unwired: 1 in, 1 out]
            n186 = property on="ButtonGoToResults" class="Bool (strict)"(error in=w254, "DisabledEnum"=w253) -> ()  [unwired: 1 in, 2 out]
          }
          event "ProcTree": Double Click {
            n187 = event-data() -> ("CtlRef"=w281:refnum<vi>, "Tag"=w276:string)  [unwired: 1 in]
            n188 = call "ProdaNG.Tree.Proc.GetTag.vi"("Tree"=w281, "Tag"=w276) -> ("Process Found"=w275:bool, "Identification"=w280:T7, "ProfInfo"=w279:string[], "SlotNo"=w272:i32)  [unwired: 5 in, 1 out]
            n189 = local write "SlotInUse"(w272) -> ()
            n190 = Select(t=T11."Enabled" ("Disabled"), s=w275, f=T11."Disabled and Grayed Out" ("Disabled")) -> (s? t:f=w267:T11)
            n191 = local write "ProfInfo"(w279) -> ()
            n192 = local write "Process Found"(w275) -> ()
            n193 = local write "Identification"(w280) -> ()
            n194 = property on="ButtonTest" class="Bool (strict)"("DisabledEnum"=w267) -> (error out=w270:errorcluster)  [unwired: 2 in, 1 out]
            n195 = local read "PrevTabState"() -> (w271:i32)
            n196 = property on="ButtonResults" class="Bool (strict)"(error in=w270, "DisabledEnum"=w267) -> (error out=w268:errorcluster)  [unwired: 1 in, 1 out]
            n197 = property on="ButtonGoToTest" class="Bool (strict)"(error in=w268, "DisabledEnum"=w267) -> (error out=w269:errorcluster)  [unwired: 1 in, 1 out]
            n198 = case shown="True" w275 {
              selector: w275 -> [_ w283]
              tunnel: w271 -> [_ w284]
              frame False {
              }
              frame True {
                n199 = case shown="Default" w284 {
                  tunnel: w283 -> [w285 w286]
                  frame Default {
                    n200 = property on="ButtonGoToTest" class="Bool (strict)"("Val(Sgnl)"=w285) -> ()  [unwired: 2 in, 2 out]
                  }
                  frame 2 {
                    n201 = property on="ButtonGoToResults" class="Bool (strict)"("Val(Sgnl)"=w286) -> ()  [unwired: 2 in, 2 out]
                  }
                }
              }
            }
            n202 = property on="ButtonGoToResults" class="Bool (strict)"(error in=w269, "DisabledEnum"=w267) -> ()  [unwired: 1 in, 2 out]
          }
          event "ProcTree": event #0x1e {
            n203 = event-data() -> ("CtlRef"=w290:refnum<vi>, "Tag"=w288:string)  [unwired: 1 in]
            n204 = call "ProdaNG.Tree.Proc.GetTag.vi"("Tree"=w290, "Tag"=w288) -> ("parent"=w287:bool, "Identification"=w289:T7)  [unwired: 5 in, 3 out]
            n205 = case shown="True" w287 {
              tunnel: w294 -> [w296 w305]
              tunnel: w293 -> [w297 w304]
              tunnel: [w296 w303] -> w292
              tunnel: [w297 w302] -> w291
              tunnel: w289 -> [_ w300]
              tunnel: w288 -> [_ w298]
              frame False {
              }
              frame True {
                n206 = Unbundle By Name(w300) -> ("WP_ID"=w299:i32)
                n207 = control-ref of="ProcTree"() -> (w301:refnum<vi>)
                n208 = call "ProdaNG.WabcoPartProcesses.Get.vi"("error in (no error)"=w305, "WabcoPartId"=w299, "dbHandleIn"=w304) -> ("error out"=w308:errorcluster, "Proc"=w306:T19[], "dbHandle"=w307:i32)  [unwired: 6 in]
                n209 = Empty Array?(array=w306) -> (empty?=w309:bool)
                n210 = case shown="False" w309 {
                  tunnel: w308 -> [w311 w333]
                  tunnel: w307 -> [w317 w334]
                  tunnel: [w316 w334] -> w302
                  tunnel: [w315 w332] -> w303
                  tunnel: w306 -> [w318 _]
                  tunnel: w301 -> [w313 w331]
                  tunnel: w299 -> [w314 _]
                  tunnel: w298 -> [w312 w330]
                  frame False {
                    n211 = call "ProdaNG.Tree.WabcoPart.Clear.vi"("Tree"=w313, "error in (no error)"=w311, "Tag"=w312) -> ("error out"=w310:errorcluster)  [unwired: 8 in]
                    n212 = for {
                      tunnel: w317 -> [w329]
                      tunnel: [w322] -> w316
                      tunnel: w318 -> [w321] mode=indexing
                      shift-right: [w323] -> w315
                      shift-left: w310 -> [w327]
                      tunnel: w313 -> [w328]
                      tunnel: w314 -> [w319]
                      n213 = call "ProdaNG.Tree.Process.Add.vi"("Tree"=w328, "error in (no error)"=w327, "WabcoPartId"=w319, "ProcessStep"=w321) -> ("error out"=w326:errorcluster)  [unwired: 7 in]
                      n214 = Unbundle By Name(w321) -> ("i_id"=w320:i32)
                      n215 = call "ProdaNG.ProcessSteps.Get.vi"("error in (no error)"=w326, "processId"=w320, "dbHandleIn"=w329) -> ("error out"=w324:errorcluster, "ProcSteps"=w325:T21[], "dbHandle"=w322:i32)  [unwired: 6 in]
                      n216 = call "ProdaNG.Tree.ProcessSteps.Add.vi"("WabcoPartId"=w319, "Tree"=w328, "error in (no error)"=w324, "ProcId"=w320, "ProcSteps in"=w325) -> ("error out"=w323:errorcluster)  [unwired: 5 in, 1 out]
                    }
                  }
                  frame True {
                    n217 = call "ProdaNG.Tree.WabcoPart.Clear.vi"("Tree"=w331, "error in (no error)"=w333, "Tag"=w330) -> ("error out"=w332:errorcluster)  [unwired: 8 in]
                  }
                }
              }
            }
          }
          event "ButtonGoToTest": Value Change {
            w343 = T11."Disabled and Grayed Out" ("Disabled")
            n218 = event-data() -> ()  [unwired: 1 in, 1 out]
            n219 = property on="ButtonGoToTest" class="Bool (strict)"("Value"=FALSE ("ButtonGoToTest")) -> ()  [unwired: 2 in, 2 out]
            n220 = local read "ProfInfo"() -> (w346:string[])
            n221 = property on="ButtonTest" class="Bool (strict)"("Val(Sgnl)"=TRUE ("Value (Signaling)")) -> (error out=w337:errorcluster)  [unwired: 2 in, 1 out]
            n222 = Array To Spreadsheet String(delimiter (Tab)=" | ", array=w346, 3:"%s" ("format string")) -> (spreadsheet string=w340:string)
            n223 = call <vilib>:"Trim Whitespace.vi"("string"=w340) -> ("trimmed string"=→"Status":string)  [unwired: 1 in]
            n224 = property on="ButtonRefreshTestTree" class="Bool (strict)"(error in=w337, "Val(Sgnl)"=TRUE ("Value (Signaling)")) -> ()  [unwired: 1 in, 2 out]
            n225 = local write "SelectedFile"(path "") -> ()
            n226 = local write "FileInUse"("") -> ()
            n227 = property on="ButtonExportFile" class="Bool (strict)"("DisabledEnum"=w343) -> ()  [unwired: 2 in, 2 out]
            n228 = local write "FileContent"(T4 {"PP"=[], "TS"=[]} ("Seq")) -> ()
            n229 = property on="ButtonCloseFile" class="Bool"("DisabledEnum"=w343) -> ()  [unwired: 2 in, 2 out]
          }
          event "ButtonGoToResults": Value Change {
            n230 = event-data() -> ()  [unwired: 1 in, 1 out]
            n231 = property on="ButtonGoToResults" class="Bool (strict)"("Value"=FALSE ("ButtonGoToResults")) -> ()  [unwired: 2 in, 2 out]
            n232 = local read "ProfInfo"() -> (w358:string[])
            n233 = property on="ButtonResults" class="Bool (strict)"("Val(Sgnl)"=TRUE ("Value (Signaling)")) -> (error out=w353:errorcluster)  [unwired: 2 in, 1 out]
            n234 = Array To Spreadsheet String(delimiter (Tab)=" | ", array=w358, 3:"%s" ("format string")) -> (spreadsheet string=w355:string)
            n235 = call <vilib>:"Trim Whitespace.vi"("string"=w355) -> ("trimmed string"=w352:string)  [unwired: 1 in]
            n236 = property on="ButtonRefreshResultTree" class="Bool (strict)"(error in=w353, "Val(Sgnl)"=TRUE ("Value (Signaling)")) -> ()  [unwired: 1 in, 2 out]
            n237 = local write "Status"(w352) -> ()
          }
          event "ButtonRefreshTestTree": Value Change {
            n238 = event-data() -> ()  [unwired: 1 in, 1 out]
            n239 = property on="TestTree" class="Tree (strict)"() -> (error out=w365:errorcluster, "Value"=w367:string[], "TopLeft"=w366:T14)  [unwired: 2 in, 1 out]
            n240 = stacked-sequence {
              tunnel: [_ _ w391 _] -> w370
              tunnel: w368 -> [_ _ w388 _]
              tunnel: w364 -> [_ _ w390 _]
              tunnel: [_ _ w389 _] -> w363
              tunnel: w367 -> [_ _ _ w414]
              tunnel: w366 -> [_ _ _ w413]
              tunnel: w365 -> [_ _ _ w412]
              tunnel: [_ _ _ w411] -> _
              frame #0 {
                w371 = TRUE ("Value (Signaling)")
                n241 = property on="ButtonRefreshTestTree" class="Bool (strict)"("Value"=w371) -> ()  [unwired: 2 in, 2 out]
                n242 = property on="Progress" class="Bool (strict)"("Visible"=w371) -> ()  [unwired: 2 in, 2 out]
                n243 = property on="Hider" class="Bool (strict)"("Visible"=w371) -> ()  [unwired: 2 in, 2 out]
              }
              frame #1 {
                n244 = local read "FPref"() -> (w372:refnum<vi>)
                n245 = property class="Pnl"(reference=w372, "DeferPanUpdts"=TRUE ("Defer Panel Updates")) -> ()  [unwired: 1 in, 2 out]
              }
              frame #2 {
                n246 = local read "Identification"() -> (w386:T7)
                n247 = local read "FileContent"() -> (w376:T4)
                n248 = control-ref of="TestTree"() -> (w387:refnum<vi>)
                n249 = call "ProdaNG.Tree.Test.Update.vi"("Identification"=w386, "FileContent"=w376, "TreeControl in"=w387, "error in (no error)"=w390, "TreeViewMode (All)"="TestTreeView", "dbHandle in"=w388) -> ("error out"=w389:errorcluster, "#changes"=w378:i32, "Number of Rows"=w380:i32, "dbHandle out"=w391:i32)  [unwired: 2 in]
                n250 = Unbundle By Name(w376) -> ("TS"=w375:T6[])
                n251 = Greater Than 0?(x=w380) -> (x > 0?=w384:bool)
                n252 = Empty Array?(array=w375) -> (empty?=w374:bool)
                n253 = Select(t=T11."Enabled" ("Disabled"), s=w384, f=T11."Disabled and Grayed Out" ("Disabled")) -> (s? t:f=w381:T11)
                n254 = property on="ButtonUnreleaseAll" class="Bool"("DisabledEnum"=w381) -> ()  [unwired: 2 in, 2 out]
                n255 = case shown="True" w374 {
                  tunnel: [w394 "No file selected"] -> w379
                  tunnel: w378 -> [w393 _]
                  tunnel: [w392 u32 13816530] -> w377
                  frame False {
                    n256 = case shown="2.." w393 {
                      selector: w393 -> [_ w398 w402]
                      tunnel: ["No changes" w400 w404] -> w394
                      tunnel: [u32 13816530 u32 16744576 u32 16744576] -> w392
                      frame Default {
                      }
                      frame 1 {
                        n257 = Format Into String(format string="%d change", w398) -> (resulting string=w400:string)  [unwired: 2 in, 1 out]
                      }
                      frame 2.. {
                        n258 = Format Into String(format string="%d changes", w402) -> (resulting string=w404:string)  [unwired: 2 in, 1 out]
                      }
                    }
                  }
                  frame True {
                  }
                }
                n259 = property on="ButtonDeleteAll" class="Bool"("DisabledEnum"=w381) -> ()  [unwired: 2 in, 2 out]
                n260 = property on="FileInUse" class="Str"("Caption.Text"=w379, "Text.BGColor"=w377) -> ()  [unwired: 2 in, 2 out]
                n261 = property on="ButtonReleaseAll" class="Bool"("DisabledEnum"=w381) -> ()  [unwired: 2 in, 2 out]
              }
              frame #3 {
                w407 = FALSE ("Value (Signaling)")
                n262 = property on="TestTree" class="Tree (strict)"(error in=w412, "Val(Sgnl)"=w414, "TopLeft"=w413) -> (error out=w411:errorcluster)  [unwired: 1 in, 1 out]
                n263 = property on="ButtonRefreshTestTree" class="Bool (strict)"("Value"=w407) -> ()  [unwired: 2 in, 2 out]
                n264 = local read "FPref"() -> (w409:refnum<vi>)
                n265 = property class="Pnl"(reference=w409, "DeferPanUpdts"=FALSE ("Defer Panel Updates")) -> ()  [unwired: 1 in, 2 out]
                n266 = property on="Progress" class="Bool (strict)"("Visible"=w407) -> ()  [unwired: 2 in, 2 out]
                n267 = property on="Hider" class="Bool (strict)"("Visible"=w407) -> ()  [unwired: 2 in, 2 out]
                n268 = local write "TestTree.OpenCloseAll"(TRUE ("TestTree.OpenCloseAll")) -> ()
              }
            }
          }
          event "TestTree": Value Change {
            n269 = event-data() -> ("CtlRef"=w427:refnum<vi>)  [unwired: 1 in]
            n270 = call "ProdaNG.Tree.Release.Get.vi"("TestStepsTree"=w427, "error in (no error)"=w444, "Release"=TRUE) -> ("error out"=w436:errorcluster, "Elements to release"=w442:T22[])  [unwired: 7 in]
            n271 = call "ProdaNG.Tree.Release.Get.vi"("TestStepsTree"=w427, "error in (no error)"=w436, "Release"=FALSE) -> ("error out"=w429:errorcluster, "Elements to release"=w432:T22[])  [unwired: 7 in]
            n272 = call "ProdaNG.Tree.Selection.GetAll.vi"("TestStepsTree"=w427, "error in (no error)"=w429) -> ("error out"=w428:errorcluster, "Selected elements"=w421:T22[])  [unwired: 7 in, 1 out]
            n273 = Array Size(array=w421) -> (size(s)=w420:i32)
            n274 = Empty Array?(array=w442) -> (empty?=w441:bool)
            n275 = Empty Array?(array=w432) -> (empty?=w433:bool)
            n276 = Empty Array?(array=w421) -> (empty?=w426:bool)
            n277 = Greater?(x=w420, y=1) -> (0:w415:bool)
            n278 = Select(t=2 ("Disabled"), s=w441, f=0 ("Disabled")) -> (s? t:f=w438:i32)
            n279 = Select(t=2 ("Disabled"), s=w433, f=0 ("Disabled")) -> (s? t:f=w431:i32)
            n280 = Select(t=2 ("Disabled"), s=w426, f=0 ("Disabled")) -> (s? t:f=w422:i32)
            n281 = Select(t=2 ("Disabled"), s=w415, f=0 ("Disabled")) -> (s? t:f=w418:i32)
            n282 = property on="ButtonRelease" class="Bool"("DisabledEnum"=w438) -> ()  [unwired: 2 in, 2 out]
            n283 = property on="ButtonUnrelease" class="Bool"("DisabledEnum"=w431) -> ()  [unwired: 2 in, 2 out]
            n284 = property on="ButtonDelete" class="Bool"("DisabledEnum"=w422) -> (error out=w423:errorcluster)  [unwired: 2 in, 1 out]
            n285 = property on="ButtonAdd" class="Bool"("DisabledEnum"=w418) -> ()  [unwired: 2 in, 2 out]
            n286 = property on="ButtonEdit" class="Bool"(error in=w423, "DisabledEnum"=w422) -> ()  [unwired: 1 in, 2 out]
          }
          event "TestTree.OpenCloseAll": Value Change {
            w452 = 0 ("Active Item:Row Number")
            n287 = event-data() -> ()  [unwired: 1 in, 1 out]
            n288 = invoke on="TestTree" class="Tree (strict)" method="Open/Close.Open/Close All"("Open"="TestTree.OpenCloseAll") -> (error out=w449:errorcluster)  [unwired: 3 in, 3 out]
            n289 = property on="ResultsTree" class="Tree (strict)"(error in=w449, "Active Item Row Number"=w452, "ActiveColNum"=w452) -> (error out=w448:errorcluster, "Active Item Tag"=w451:string)  [unwired: 1 in, 1 out]
            n290 = Bundle By Name(cluster=T14 {"Node"="", "Column"=0} ("Top Left Visible Cell"), "Node"=w451) -> (w447:T14)
            n291 = property on="ResultsTree" class="Tree (strict)"(error in=w448, "TopLeft"=w447) -> (error out=w446:errorcluster)  [unwired: 1 in, 1 out]
            n292 = Unbundle(w446) -> ()  [unwired: 3 out]
          }
          event "ButtonRelease": Value Change {
            w461 = TRUE ("Release")
            n293 = event-data() -> ()  [unwired: 1 in, 1 out]
            n294 = control-ref of="TestTree"() -> (w462:refnum<vi>)
            n295 = call "ProdaNG.Tree.Release.Get.vi"("TestStepsTree"=w462, "error in (no error)"=w463, "Release"=w461) -> ("error out"=w458:errorcluster, "Elements to release"=w460:T22[])  [unwired: 7 in]
            n296 = Empty Array?(array=w460) -> (empty?=w459:bool)
            n297 = case shown="False" w459 {
              tunnel: w466 -> [w476 w500]
              tunnel: [w475 w499] -> w465
              tunnel: [w474 w500] -> w464
              tunnel: w458 -> [w473 w499]
              tunnel: w462 -> [w472 _]
              tunnel: w461 -> [w471 _]
              tunnel: w460 -> [w470 _]
              tunnel: w457 -> [w467 _]
              frame False {
                n298 = call "ProdaNG.Configurator.Popup.Release.vi"("Release"=w471, "Elements to release/unrelease"=w470) -> ("Reason out"=w469:string, "OK?"=w468:bool)  [unwired: 8 in]
                n299 = case shown="\"ProcessFound\"" w467 {
                  tunnel: w476 -> [w478 w487]
                  tunnel: [w477 w486] -> w475
                  tunnel: [w478 w485] -> w474
                  tunnel: w473 -> [w477 w484]
                  tunnel: w472 -> [_ w483]
                  tunnel: w471 -> [_ w482]
                  tunnel: w470 -> [_ w481]
                  tunnel: w469 -> [_ w480]
                  tunnel: w468 -> [_ w479]
                  frame Default {
                  }
                  frame "ProcessFound" {
                    n300 = case shown="True" w479 {
                      tunnel: w487 -> [w489 w498]
                      tunnel: [w488 w497] -> w486
                      tunnel: [w489 w496] -> w485
                      tunnel: w484 -> [w488 w495]
                      tunnel: w483 -> [_ w494]
                      tunnel: w481 -> [_ w493]
                      tunnel: w482 -> [_ w492]
                      tunnel: w480 -> [_ w490]
                      frame False {
                      }
                      frame True {
                        n301 = property on="ButtonRefreshTestTree" class="Bool (strict)"("Val(Sgnl)"=TRUE ("Value (Signaling)")) -> ()  [unwired: 2 in, 2 out]
                        n302 = call "ProdaNG.Tree.Release.vi"("comment"=w490, "TestStepsTree"=w494, "error in (no error)"=w495, "Release"=w492, "Elements to release/unrelease"=w493, "dbHandleIn"=w498) -> ("error out"=w497:errorcluster, "dbHandle"=w496:i32)  [unwired: 4 in]
                      }
                    }
                  }
                }
              }
              frame True {
              }
            }
          }
          event "ButtonReleaseAll": Value Change {
            w505 = TRUE ("Release")
            n303 = event-data() -> ()  [unwired: 1 in, 1 out]
            n304 = control-ref of="TestTree"() -> (w506:refnum<vi>)
            n305 = call "ProdaNG.Tree.Release.GetAll.vi"("TestStepsTree"=w506, "error in (no error)"=w507, "Release"=w505) -> ("error out"=w502:errorcluster, "Elements to release"=w504:T22[])  [unwired: 7 in]
            n306 = Empty Array?(array=w504) -> (empty?=w503:bool)
            n307 = case shown="False" w503 {
              tunnel: w510 -> [w520 w544]
              tunnel: [w519 w543] -> w509
              tunnel: [w518 w544] -> w508
              tunnel: w502 -> [w517 w543]
              tunnel: w506 -> [w516 _]
              tunnel: w505 -> [w515 _]
              tunnel: w504 -> [w514 _]
              tunnel: w501 -> [w511 _]
              frame False {
                n308 = call "ProdaNG.Configurator.Popup.Release.vi"("Release"=w515, "Elements to release/unrelease"=w514) -> ("Reason out"=w513:string, "OK?"=w512:bool)  [unwired: 8 in]
                n309 = case shown="\"ProcessFound\"" w511 {
                  tunnel: w520 -> [w522 w531]
                  tunnel: [w521 w530] -> w519
                  tunnel: [w522 w529] -> w518
                  tunnel: w517 -> [w521 w528]
                  tunnel: w516 -> [_ w527]
                  tunnel: w515 -> [_ w526]
                  tunnel: w514 -> [_ w525]
                  tunnel: w513 -> [_ w524]
                  tunnel: w512 -> [_ w523]
                  frame Default {
                  }
                  frame "ProcessFound" {
                    n310 = case shown="True" w523 {
                      tunnel: w531 -> [w533 w542]
                      tunnel: [w532 w541] -> w530
                      tunnel: [w533 w540] -> w529
                      tunnel: w528 -> [w532 w539]
                      tunnel: w527 -> [_ w538]
                      tunnel: w525 -> [_ w537]
                      tunnel: w526 -> [_ w536]
                      tunnel: w524 -> [_ w534]
                      frame False {
                      }
                      frame True {
                        n311 = property on="ButtonRefreshTestTree" class="Bool (strict)"("Val(Sgnl)"=TRUE ("Value (Signaling)")) -> ()  [unwired: 2 in, 2 out]
                        n312 = call "ProdaNG.Tree.Release.vi"("comment"=w534, "TestStepsTree"=w538, "error in (no error)"=w539, "Release"=w536, "Elements to release/unrelease"=w537, "dbHandleIn"=w542) -> ("error out"=w541:errorcluster, "dbHandle"=w540:i32)  [unwired: 4 in]
                      }
                    }
                  }
                }
              }
              frame True {
              }
            }
          }
          event "ButtonUnrelease": Value Change {
            w549 = FALSE ("Release")
            n313 = event-data() -> ()  [unwired: 1 in, 1 out]
            n314 = control-ref of="TestTree"() -> (w550:refnum<vi>)
            n315 = call "ProdaNG.Tree.Release.Get.vi"("TestStepsTree"=w550, "error in (no error)"=w551, "Release"=w549) -> ("error out"=w546:errorcluster, "Elements to release"=w548:T22[])  [unwired: 7 in]
            n316 = Empty Array?(array=w548) -> (empty?=w547:bool)
            n317 = case shown="False" w547 {
              tunnel: w554 -> [w564 w588]
              tunnel: [w563 w587] -> w553
              tunnel: [w562 w588] -> w552
              tunnel: w546 -> [w561 w587]
              tunnel: w550 -> [w560 _]
              tunnel: w549 -> [w559 _]
              tunnel: w548 -> [w558 _]
              tunnel: w545 -> [w555 _]
              frame False {
                n318 = call "ProdaNG.Configurator.Popup.Release.vi"("Release"=w559, "Elements to release/unrelease"=w558) -> ("Reason out"=w557:string, "OK?"=w556:bool)  [unwired: 8 in]
                n319 = case shown="\"ProcessFound\"" w555 {
                  tunnel: w564 -> [w566 w575]
                  tunnel: [w565 w574] -> w563
                  tunnel: [w566 w573] -> w562
                  tunnel: w561 -> [w565 w572]
                  tunnel: w560 -> [_ w571]
                  tunnel: w559 -> [_ w570]
                  tunnel: w558 -> [_ w569]
                  tunnel: w557 -> [_ w568]
                  tunnel: w556 -> [_ w567]
                  frame Default {
                  }
                  frame "ProcessFound" {
                    n320 = case shown="True" w567 {
                      tunnel: w575 -> [w577 w586]
                      tunnel: [w576 w585] -> w574
                      tunnel: [w577 w584] -> w573
                      tunnel: w572 -> [w576 w583]
                      tunnel: w571 -> [_ w582]
                      tunnel: w569 -> [_ w581]
                      tunnel: w570 -> [_ w580]
                      tunnel: w568 -> [_ w578]
                      frame False {
                      }
                      frame True {
                        n321 = property on="ButtonRefreshTestTree" class="Bool (strict)"("Val(Sgnl)"=TRUE ("Value (Signaling)")) -> ()  [unwired: 2 in, 2 out]
                        n322 = call "ProdaNG.Tree.Release.vi"("comment"=w578, "TestStepsTree"=w582, "error in (no error)"=w583, "Release"=w580, "Elements to release/unrelease"=w581, "dbHandleIn"=w586) -> ("error out"=w585:errorcluster, "dbHandle"=w584:i32)  [unwired: 4 in]
                      }
                    }
                  }
                }
              }
              frame True {
              }
            }
          }
          event "ButtonUnreleaseAll": Value Change {
            w593 = FALSE ("Release")
            n323 = event-data() -> ()  [unwired: 1 in, 1 out]
            n324 = control-ref of="TestTree"() -> (w594:refnum<vi>)
            n325 = call "ProdaNG.Tree.Release.GetAll.vi"("TestStepsTree"=w594, "error in (no error)"=w595, "Release"=w593) -> ("error out"=w590:errorcluster, "Elements to release"=w592:T22[])  [unwired: 7 in]
            n326 = Empty Array?(array=w592) -> (empty?=w591:bool)
            n327 = case shown="False" w591 {
              tunnel: w598 -> [w608 w632]
              tunnel: [w607 w631] -> w597
              tunnel: [w606 w632] -> w596
              tunnel: w590 -> [w605 w631]
              tunnel: w594 -> [w604 _]
              tunnel: w593 -> [w603 _]
              tunnel: w592 -> [w602 _]
              tunnel: w589 -> [w599 _]
              frame False {
                n328 = call "ProdaNG.Configurator.Popup.Release.vi"("Release"=w603, "Elements to release/unrelease"=w602) -> ("Reason out"=w601:string, "OK?"=w600:bool)  [unwired: 8 in]
                n329 = case shown="\"ProcessFound\"" w599 {
                  tunnel: w608 -> [w610 w619]
                  tunnel: [w609 w618] -> w607
                  tunnel: [w610 w617] -> w606
                  tunnel: w605 -> [w609 w616]
                  tunnel: w604 -> [_ w615]
                  tunnel: w603 -> [_ w614]
                  tunnel: w602 -> [_ w613]
                  tunnel: w601 -> [_ w612]
                  tunnel: w600 -> [_ w611]
                  frame Default {
                  }
                  frame "ProcessFound" {
                    n330 = case shown="True" w611 {
                      tunnel: w619 -> [w621 w630]
                      tunnel: [w620 w629] -> w618
                      tunnel: [w621 w628] -> w617
                      tunnel: w616 -> [w620 w627]
                      tunnel: w615 -> [_ w626]
                      tunnel: w613 -> [_ w625]
                      tunnel: w614 -> [_ w624]
                      tunnel: w612 -> [_ w622]
                      frame False {
                      }
                      frame True {
                        n331 = property on="ButtonRefreshTestTree" class="Bool (strict)"("Val(Sgnl)"=TRUE ("Value (Signaling)")) -> ()  [unwired: 2 in, 2 out]
                        n332 = call "ProdaNG.Tree.Release.vi"("comment"=w622, "TestStepsTree"=w626, "error in (no error)"=w627, "Release"=w624, "Elements to release/unrelease"=w625, "dbHandleIn"=w630) -> ("error out"=w629:errorcluster, "dbHandle"=w628:i32)  [unwired: 4 in]
                      }
                    }
                  }
                }
              }
              frame True {
              }
            }
          }
          event "ButtonAdd": Value Change {
            n333 = event-data() -> ()  [unwired: 1 in, 1 out]
            n334 = control-ref of="TestTree"() -> (w648:refnum<vi>)
            n335 = call "ProdaNG.Units.Get.vi"("error in (no error)"=w638, "dbHandleIn"=w637) -> ("error out"=w636:errorcluster, "units simple"=w634:T24[], "dbHandle"=w635:i32)  [unwired: 6 in, 1 out]
            n336 = call "ProdaNG.Tree.Selection.GetTS.vi"("TestStepsTree"=w648, "error in (no error)"=w636) -> ("error out"=w646:errorcluster, "LastTS"=w647:T22)  [unwired: 8 in]
            n337 = local read "Identification"() -> (w639:T7)
            n338 = call "ProdaNG.Configurator.Popup.Add.vi"("units simple"=w634, "Selected element"=w647) -> ("Selected elements value out"=w641:T5, "Selected element out"=w633:T22, "Reason out"=w640:string, "OK?"=w642:bool)  [unwired: 6 in]
            n339 = case shown="\"ProcessFound\"" w643 {
              tunnel: w635 -> [w649 w660]
              tunnel: [w650 w659] -> w645
              tunnel: [w649 w658] -> w644
              tunnel: w646 -> [w650 w657]
              tunnel: w648 -> [_ w656]
              tunnel: w633 -> [_ w655]
              tunnel: w642 -> [_ w654]
              tunnel: w641 -> [_ w653]
              tunnel: w640 -> [_ w652]
              tunnel: w639 -> [_ w651]
              frame Default {
              }
              frame "ProcessFound" {
                n340 = case shown="True" w654 {
                  tunnel: w660 -> [w662 w672]
                  tunnel: [w661 w671] -> w659
                  tunnel: [w662 w670] -> w658
                  tunnel: w657 -> [w661 w669]
                  tunnel: w656 -> [_ w668]
                  tunnel: w655 -> [_ w667]
                  tunnel: w653 -> [_ w664]
                  tunnel: w652 -> [_ w665]
                  tunnel: w651 -> [_ w663]
                  frame False {
                  }
                  frame True {
                    n341 = property on="ButtonRefreshTestTree" class="Bool (strict)"("Val(Sgnl)"=TRUE ("Value (Signaling)")) -> ()  [unwired: 2 in, 2 out]
                    n342 = call "ProdaNG.Tree.Add.vi"("Identification"=w663, "reason"=w665, "TestStepsTree"=w668, "error in (no error)"=w669, "Element values"=w664, "Element to add"=w667, "dbHandleIn"=w672) -> ("error out"=w671:errorcluster, "dbHandle"=w670:i32)  [unwired: 3 in]
                  }
                }
              }
            }
          }
          event "ButtonEdit": Value Change; "TestTree": Double Click {
            n343 = event-data() -> ()  [unwired: 1 in, 1 out]
            n344 = control-ref of="TestTree"() -> (w685:refnum<vi>)
            n345 = call "ProdaNG.Units.Get.vi"("error in (no error)"=w677, "dbHandleIn"=w674) -> ("error out"=w676:errorcluster, "units simple"=w673:T24[], "dbHandle"=w675:i32)  [unwired: 6 in, 1 out]
            n346 = call "ProdaNG.Tree.Selection.GetAll.vi"("TestStepsTree"=w685, "error in (no error)"=w676) -> ("error out"=w682:errorcluster, "Selected elements values"=w678:T5[], "Selected elements"=w684:T22[])  [unwired: 7 in]
            n347 = Empty Array?(array=w684) -> (empty?=w683:bool)
            n348 = case shown="False" w683 {
              tunnel: w675 -> [w697 w721]
              tunnel: [w696 w720] -> w681
              tunnel: [w695 w721] -> w680
              tunnel: w682 -> [w694 w720]
              tunnel: w685 -> [w693 _]
              tunnel: w684 -> [w692 _]
              tunnel: w679 -> [w690 _]
              tunnel: w678 -> [w689 _]
              tunnel: w673 -> [w686 _]
              frame False {
                n349 = call "ProdaNG.Configurator.Popup.Edit.vi"("units simple"=w686, "Selected elements values"=w689, "Elements to edit"=w692) -> ("Selected elements values out"=w688:T5[], "Reason out"=w687:string, "OK?"=w691:bool)  [unwired: 6 in]
                n350 = case shown="\"ProcessFound\"" w690 {
                  tunnel: w697 -> [w698 w708]
                  tunnel: [w699 w707] -> w696
                  tunnel: [w698 w706] -> w695
                  tunnel: w694 -> [w699 w705]
                  tunnel: w693 -> [_ w704]
                  tunnel: w692 -> [_ w703]
                  tunnel: w691 -> [_ w702]
                  tunnel: w688 -> [_ w701]
                  tunnel: w687 -> [_ w700]
                  frame Default {
                  }
                  frame "ProcessFound" {
                    n351 = case shown="True" w702 {
                      tunnel: w708 -> [w710 w719]
                      tunnel: [w709 w718] -> w707
                      tunnel: [w710 w717] -> w706
                      tunnel: w705 -> [w709 w716]
                      tunnel: w704 -> [_ w715]
                      tunnel: w703 -> [_ w714]
                      tunnel: w701 -> [_ w712]
                      tunnel: w700 -> [_ w713]
                      frame False {
                      }
                      frame True {
                        n352 = property on="ButtonRefreshTestTree" class="Bool (strict)"("Val(Sgnl)"=TRUE ("Value (Signaling)")) -> ()  [unwired: 2 in, 2 out]
                        n353 = call "ProdaNG.Tree.Edit.vi"("reason"=w713, "TestStepsTree"=w715, "error in (no error)"=w716, "Selected elements values"=w712, "Selected elements"=w714, "dbHandleIn"=w719) -> ("error out"=w718:errorcluster, "dbHandle"=w717:i32)  [unwired: 4 in]
                      }
                    }
                  }
                }
              }
              frame True {
              }
            }
          }
          event "ButtonDelete": Value Change {
            n354 = event-data() -> ()  [unwired: 1 in, 1 out]
            n355 = control-ref of="TestTree"() -> (w730:refnum<vi>)
            n356 = call "ProdaNG.Tree.Selection.GetAll.vi"("TestStepsTree"=w730, "error in (no error)"=w726) -> ("error out"=w727:errorcluster, "Selected elements"=w729:T22[])  [unwired: 7 in, 1 out]
            n357 = Empty Array?(array=w729) -> (empty?=w728:bool)
            n358 = case shown="False" w728 {
              tunnel: w725 -> [w738 w758]
              tunnel: [w737 w757] -> w724
              tunnel: [w736 w758] -> w723
              tunnel: w727 -> [w735 w757]
              tunnel: w730 -> [w734 _]
              tunnel: w729 -> [w733 _]
              tunnel: w722 -> [w731 _]
              frame False {
                n359 = call "ProdaNG.Configurator.Popup.Delete.vi"("Elements to delete"=w733) -> ("OK?"=w732:bool)  [unwired: 10 in]
                n360 = case shown="\"ProcessFound\"" w731 {
                  tunnel: w738 -> [w739 w747]
                  tunnel: [w740 w746] -> w737
                  tunnel: [w739 w745] -> w736
                  tunnel: w735 -> [w740 w744]
                  tunnel: w734 -> [_ w743]
                  tunnel: w733 -> [_ w742]
                  tunnel: w732 -> [_ w741]
                  frame Default {
                  }
                  frame "ProcessFound" {
                    n361 = case shown="True" w741 {
                      tunnel: w747 -> [w749 w756]
                      tunnel: [w748 w755] -> w746
                      tunnel: [w749 w754] -> w745
                      tunnel: w744 -> [w748 w753]
                      tunnel: w743 -> [_ w752]
                      tunnel: w742 -> [_ w751]
                      frame False {
                      }
                      frame True {
                        n362 = property on="ButtonRefreshTestTree" class="Bool (strict)"("Val(Sgnl)"=TRUE ("Value (Signaling)")) -> ()  [unwired: 2 in, 2 out]
                        n363 = call "ProdaNG.Tree.Delete.vi"("TestStepsTree"=w752, "error in (no error)"=w753, "Elements to delete"=w751, "dbHandleIn"=w756) -> ("error out"=w755:errorcluster, "dbHandle"=w754:i32)  [unwired: 6 in]
                      }
                    }
                  }
                }
              }
              frame True {
              }
            }
          }
          event "ButtonDeleteAll": Value Change {
            n364 = event-data() -> ()  [unwired: 1 in, 1 out]
            n365 = control-ref of="TestTree"() -> (w767:refnum<vi>)
            n366 = call "ProdaNG.Tree.GetAll.vi"("TestStepsTree"=w767, "error in (no error)"=w763) -> ("error out"=w764:errorcluster, "Selected elements"=w766:T22[])  [unwired: 7 in, 1 out]
            n367 = Empty Array?(array=w766) -> (empty?=w765:bool)
            n368 = case shown="False" w765 {
              tunnel: w762 -> [w775 w795]
              tunnel: [w774 w794] -> w761
              tunnel: [w773 w795] -> w760
              tunnel: w764 -> [w772 w794]
              tunnel: w767 -> [w771 _]
              tunnel: w766 -> [w770 _]
              tunnel: w759 -> [w768 _]
              frame False {
                n369 = call "ProdaNG.Configurator.Popup.Delete.vi"("Elements to delete"=w770) -> ("OK?"=w769:bool)  [unwired: 10 in]
                n370 = case shown="\"ProcessFound\"" w768 {
                  tunnel: w775 -> [w776 w784]
                  tunnel: [w777 w783] -> w774
                  tunnel: [w776 w782] -> w773
                  tunnel: w772 -> [w777 w781]
                  tunnel: w771 -> [_ w780]
                  tunnel: w770 -> [_ w779]
                  tunnel: w769 -> [_ w778]
                  frame Default {
                  }
                  frame "ProcessFound" {
                    n371 = case shown="True" w778 {
                      tunnel: w784 -> [w786 w793]
                      tunnel: [w785 w792] -> w783
                      tunnel: [w786 w791] -> w782
                      tunnel: w781 -> [w785 w790]
                      tunnel: w780 -> [_ w789]
                      tunnel: w779 -> [_ w788]
                      frame False {
                      }
                      frame True {
                        n372 = property on="ButtonRefreshTestTree" class="Bool (strict)"("Val(Sgnl)"=TRUE ("Value (Signaling)")) -> ()  [unwired: 2 in, 2 out]
                        n373 = call "ProdaNG.Tree.Delete.vi"("TestStepsTree"=w789, "error in (no error)"=w790, "Elements to delete"=w788, "dbHandleIn"=w793) -> ("error out"=w792:errorcluster, "dbHandle"=w791:i32)  [unwired: 6 in]
                      }
                    }
                  }
                }
              }
              frame True {
              }
            }
          }
          event "ButtonOpenFile": Value Change {
            n374 = event-data() -> ()  [unwired: 1 in, 1 out]
            n375 = local read "SelectedFile"() -> (w797:path)
            n376 = call "File exists.vi"("file path"=w797) -> ("exists?"=w798:bool)  [unwired: 4 in]
            n377 = case shown="True" w798 {
              tunnel: [w813 TRUE] -> w804
              tunnel: [w810 w816] -> w803
              tunnel: w802 -> [w808 w815]
              tunnel: [w807 w815] -> w800
              tunnel: w797 -> [_ w816]
              frame False {
                n378 = call "File Dialog2"("prompt"="Select seqeunce configuration flie...", "error in"=w808, "pattern (all files)"="*.ini") -> ("selected path"=w810:path, "exists"=w806:bool, "cancelled"=w811:bool, "error out"=w807:errorcluster)  [unwired: 9 in]
                n379 = Compound Arithmetic op=AND(w806, invert w811) -> (w813:bool)
              }
              frame True {
              }
            }
            n380 = case shown="True" w804 {
              tunnel: w800 -> [w818 w827]
              tunnel: w803 -> [_ w824]
              tunnel: [w817 w821] -> w801
              tunnel: w799 -> [_ w828]
              frame False {
                n381 = call <vilib>:"Clear Errors.vi"("error in (no error)"=w818) -> ("error out"=w817:errorcluster)  [unwired: 5 in, 1 out]
              }
              frame True {
                n382 = local read "SlotInUse"() -> (w819:i32)
                n383 = call "ProdaNG.Units.Get.vi"("error in (no error)"=w827, "dbHandleIn"=w828) -> ("error out"=w826:errorcluster, "units simple"=w825:T24[])  [unwired: 6 in, 2 out]
                n384 = call "ProdaNG.File.Read.vi"("Config"="Configuration", "error in (no error)"=w826, "units"=w825, "SeqFile Path"=w824, "SlotNo"=w819) -> ("error out"=w821:errorcluster, "Seq"=w822:T4)  [unwired: 4 in, 1 out]
                n385 = call <vilib>:"Get File Extension.vi"("file"=w824) -> ("filename without extension"=w823:string)  [unwired: 6 in, 4 out]
                n386 = case shown="No Error" w821 {
                  tunnel: w823 -> [w840 _]
                  tunnel: w822 -> [w835 _]
                  tunnel: w819 -> [w833 _]
                  frame No Error {
                    w843 = T11."Enabled" ("Disabled")
                    n387 = property on="ButtonRefreshTestTree" class="Bool (strict)"("Val(Sgnl)"=TRUE ("Value (Signaling)")) -> ()  [unwired: 2 in, 2 out]
                    n388 = Compound Arithmetic op=ADD(w833, 65 ("value")) -> (w842:i32)
                    n389 = Build Array(w842) -> (w839:i32[])
                    n390 = Greater Or Equal To 0?(x=w833) -> (x >= 0?=w832:bool)
                    n391 = Byte Array To String(unsigned byte array=w839) -> (string=w834:string)
                    n392 = property on="ButtonExportFile" class="Bool (strict)"("DisabledEnum"=w843) -> ()  [unwired: 2 in, 2 out]
                    n393 = Select(t=w834, s=w832, f="") -> (s? t:f=w830:string)
                    n394 = Format Into String(format string="%s %s", w840, w830) -> (resulting string=w837:string)  [unwired: 2 in, 1 out]
                    n395 = property on="ButtonCloseFile" class="Bool"("DisabledEnum"=w843) -> ()  [unwired: 2 in, 2 out]
                    n396 = call <vilib>:"Trim Whitespace.vi"("string"=w837) -> ("trimmed string"=→"FileInUse":string)  [unwired: 1 in]
                    n397 = property on="FileInUse" class="Str"("Text.BGColor"=u32 13816530) -> ()  [unwired: 2 in, 2 out]
                    "FileContent" <- w835
                  }
                  frame Error {
                  }
                }
                "SelectedFile" <- w824
              }
            }
            n398 = property on="ButtonOpenFile" class="Bool (strict)"("Value"=FALSE ("ButtonOpenFile")) -> ()  [unwired: 2 in, 2 out]
          }
          event "ButtonCloseFile": Value Change {
            w847 = T11."Disabled and Grayed Out" ("Disabled")
            n399 = event-data() -> ()  [unwired: 1 in, 1 out]
            n400 = property on="ButtonExportFile" class="Bool (strict)"("DisabledEnum"=w847) -> ()  [unwired: 2 in, 2 out]
            n401 = local write "FileContent"(T4 {"PP"=[], "TS"=[]} ("Seq")) -> ()
            n402 = local write "SelectedFile"(path "" ("SelectedFile")) -> ()
            n403 = local write "FileInUse"("") -> ()
            n404 = property on="ButtonCloseFile" class="Bool"("DisabledEnum"=w847) -> ()  [unwired: 2 in, 2 out]
            n405 = property on="ButtonRefreshTestTree" class="Bool (strict)"("Val(Sgnl)"=TRUE ("Value (Signaling)")) -> ()  [unwired: 2 in, 2 out]
          }
          event "ButtonExportFile": Value Change {
            n406 = event-data() -> ()  [unwired: 1 in, 1 out]
            n407 = Two Button Dialog(message="Data will be exported to production database!!!\n\n Do you want to continue?") -> (T button?=w854:bool)  [unwired: 2 in]
            n408 = case shown="True" w854 {
              tunnel: w858 -> [w861 w866]
              tunnel: w857 -> [w860 w865]
              tunnel: [w861 w864] -> w856
              tunnel: [w860 w863] -> w855
              frame False {
                n409 = property on="ButtonExportFile" class="Bool (strict)"("Value"=FALSE ("ButtonExportFile")) -> ()  [unwired: 2 in, 2 out]
              }
              frame True {
                n410 = stacked-sequence {
                  tunnel: w866 -> [_ w877 _]
                  tunnel: w865 -> [_ w876 _]
                  tunnel: [_ w872 _] -> w864
                  tunnel: [_ w871 _] -> w863
                  frame #0 {
                    w867 = TRUE ("Visible")
                    n411 = local read "FPref"() -> (w868:refnum<vi>)
                    n412 = property on="Hider" class="Bool (strict)"("Visible"=w867) -> ()  [unwired: 2 in, 2 out]
                    n413 = property on="Progress" class="Bool (strict)"("Visible"=w867) -> ()  [unwired: 2 in, 2 out]
                    n414 = property class="Pnl"(reference=w868, "DeferPanUpdts"=TRUE ("Defer Panel Updates")) -> ()  [unwired: 1 in, 2 out]
                  }
                  frame #1 {
                    n415 = local read "Identification"() -> (w870:T7)
                    n416 = local read "FileContent"() -> (w874:T4)
                    n417 = control-ref of="TestTree"() -> (w875:refnum<vi>)
                    n418 = call "ProdaNG.File.ExportToDB.vi"("Identification"=w870, "reason"="Exported by Proda Configurator", "TestStepsTree"=w875, "error in (no error)"=w876, "FileContent"=w874, "dbHandleIn"=w877) -> ("error out"=w871:errorcluster, "dbHandle"=w872:i32)  [unwired: 4 in]
                  }
                  frame #2 {
                    w878 = FALSE ("Visible")
                    n419 = local read "FPref"() -> (w881:refnum<vi>)
                    n420 = property on="ButtonExportFile" class="Bool (strict)"("Value"=FALSE ("ButtonExportFile")) -> ()  [unwired: 2 in, 2 out]
                    n421 = property on="Hider" class="Bool (strict)"("Visible"=w878) -> ()  [unwired: 2 in, 2 out]
                    n422 = property class="Pnl"(reference=w881, "DeferPanUpdts"=FALSE ("Defer Panel Updates")) -> ()  [unwired: 1 in, 2 out]
                    n423 = property on="Progress" class="Bool (strict)"("Visible"=w878) -> ()  [unwired: 2 in, 2 out]
                    n424 = property on="ButtonRefreshTestTree" class="Bool (strict)"("Val(Sgnl)"=TRUE ("Value (Signaling)")) -> ()  [unwired: 2 in, 2 out]
                  }
                }
              }
            }
          }
          event "ButtonSaveToFile": Value Change {
            n425 = event-data() -> ()  [unwired: 1 in, 1 out]
            n426 = local read "ProfInfo"() -> (w883:string[])
            n427 = local read "SelectedFile"() -> (w897:path)
            n428 = call "File exists.vi"("file path"=w897) -> ("exists?"=w898:bool)  [unwired: 4 in]
            n429 = Index Array(array=w883) -> (element=w891:string)  [unwired: 1 in]
            n430 = call <vilib>:"Space Constant.vi"() -> ("String"=w889:string)
            n431 = call "ProdaNG.Units.Get.vi"("error in (no error)"=w887, "dbHandleIn"=w888) -> ("error out"=w885:errorcluster, "units simple"=w884:T24[], "dbHandle"=w886:i32)  [unwired: 6 in, 1 out]
            n432 = Match Pattern(string=w891, regular expression=w889) -> (before substring=w890:string)  [unwired: 1 in, 3 out]
            n433 = Concatenate Strings(w890, ".ini" ("string")) -> (w893:string)
            n434 = case shown="False" w898 {
              tunnel: w897 -> [_ w910]
              tunnel: [w905 w910] -> w896
              tunnel: [w904 w908] -> w895
              tunnel: w893 -> [w901 _]
              tunnel: [w903 w912] -> w892
              tunnel: w885 -> [w902 w912]
              frame False {
                n435 = call "File Dialog"("prompt"="Select seqeunce configuration flie...", "default name"=w901, "error in"=w902, "pattern (all files)"="*.ini") -> ("selected path"=w905:path, "cancelled"=w904:bool, "error out"=w903:errorcluster)  [unwired: 8 in, 1 out]
              }
              frame True {
                n436 = Two Button Dialog(message="File will be overwritten. Do you want to continue?") -> (T button?=w909:bool)  [unwired: 2 in]
                n437 = Not(x=w909) -> (.not. x?=w908:bool)
              }
            }
            n438 = case shown="False" w895 {
              tunnel: w892 -> [w920 w923]
              tunnel: [w922 w923] -> w899
              tunnel: w896 -> [w915 _]
              tunnel: w884 -> [w914 _]
              tunnel: w883 -> [w913 _]
              frame False {
                n439 = call "ProdaNG.File.ExportToFile.vi"("error in (no error)"=w920) -> ("error out"=w919:errorcluster, "FileContent"=w918:T4)  [unwired: 9 in]
                n440 = local write "SelectedFile"(w915) -> ()
                n441 = local read "Configuration"() -> (w917:T8)
                n442 = local write "FileContent"(w918) -> ()
                n443 = property on="ButtonOpenFile" class="Bool (strict)"("Val(Sgnl)"=TRUE ("ButtonOpenFile")) -> ()  [unwired: 2 in, 2 out]
                n444 = local read "SlotInUse"() -> (w921:i32)
                n445 = call "ProdaNG.File.Write.vi"("ProfInfo"=w913, "Config"=w917, "SlotNo"=w921, "error in (no error)"=w919, "units"=w914, "Seq"=w918, "SeqFile Path"=w915) -> ("error out"=w922:errorcluster)  [unwired: 4 in]
              }
              frame True {
              }
            }
          }
          event "ButtonRefreshResultTree": Value Change {
            n446 = event-data() -> ()  [unwired: 1 in, 1 out]
            n447 = property on="ResultsTree" class="Tree (strict)"() -> (error out=w926:errorcluster, "Value"=w928:string[], "TopLeft"=w927:T14)  [unwired: 2 in, 1 out]
            n448 = stacked-sequence {
              tunnel: [_ _ _ w987 _] -> w931
              tunnel: w929 -> [_ _ _ w981 _]
              tunnel: w925 -> [_ _ _ w982 _]
              tunnel: [_ _ _ w985 _] -> w924
              tunnel: w928 -> [_ _ _ _ w1005]
              tunnel: w927 -> [_ _ _ _ w1004]
              tunnel: w926 -> [_ _ _ _ w1003]
              tunnel: [_ _ _ _ w1002] -> _
              frame #0 {
                w932 = TRUE ("Value (Signaling)")
                n449 = property on="ButtonRefreshResultTree" class="Bool (strict)"("Value"=w932) -> ()  [unwired: 2 in, 2 out]
                n450 = property on="Progress" class="Bool (strict)"("Visible"=w932) -> ()  [unwired: 2 in, 2 out]
                n451 = property on="Hider" class="Bool (strict)"("Visible"=w932) -> ()  [unwired: 2 in, 2 out]
              }
              frame #1 {
                n452 = local read "FPref"() -> (w933:refnum<vi>)
                n453 = property class="Pnl"(reference=w933, "DeferPanUpdts"=TRUE ("Defer Panel Updates")) -> ()  [unwired: 1 in, 2 out]
              }
              frame #2 {
                n454 = local read "DBtime"() -> (w937:timestamp)
                n455 = case shown="\"Custom\"" "ResultsSpan" {
                  tunnel: [w941 w945 w951 w956 w961 w966] -> w939
                  tunnel: w937 -> [_ w946 w951 w956 w961 w966]
                  tunnel: [w940 w942 w952 w957 w962 w967] -> w936
                  tunnel: "ResultsAmount" -> [_ w944 w950 w955 w960 w965]
                  frame "Custom" {
                    n456 = local read "Results.TimeFrom"() -> (w940:timestamp)
                    n457 = local read "Results.TimeTo"() -> (w941:timestamp)
                  }
                  frame "Shift(s)" {
                    n458 = call "GetShiftTime.vi"("Time"=w946) -> ("Shift End Time"=w945:timestamp)  [unwired: 7 in, 3 out]
                    n459 = Compound Arithmetic op=MULTIPLY(w944, 28800) -> (w943:i32)
                    n460 = Subtract(x=w945, y=w943) -> (x-y=w942:timestamp)
                  }
                  frame "Hour(s)" {
                    n461 = Compound Arithmetic op=MULTIPLY(w950, 3600) -> (w949:i32)
                    n462 = Subtract(x=w951, y=w949) -> (x-y=w952:timestamp)
                  }
                  frame "Day(s)" {
                    n463 = Compound Arithmetic op=MULTIPLY(w955, 86400) -> (w954:i32)
                    n464 = Subtract(x=w956, y=w954) -> (x-y=w957:timestamp)
                  }
                  frame "Week(s)" {
                    n465 = Compound Arithmetic op=MULTIPLY(w960, 604800) -> (w959:i32)
                    n466 = Subtract(x=w961, y=w959) -> (x-y=w962:timestamp)
                  }
                  frame "Month(s)" {
                    n467 = Compound Arithmetic op=MULTIPLY(w965, 2592000) -> (w964:i32)
                    n468 = Subtract(x=w966, y=w964) -> (x-y=w967:timestamp)
                  }
                }
                n469 = local write "Results.TimeTo"(w939) -> ()
                n470 = local write "Results.TimeFrom"(w936) -> ()
              }
              frame #3 {
                w978 = "%d.%m.%Y %H:%M:%S" ("time format string")
                n471 = local read "Identification"() -> (w988:T7)
                n472 = property on="ProductList" class="LstBox (strict)"(error in=w982) -> (error out=w989:errorcluster, "Item Names"=w991:string[], "Value"=w990:i32[])  [unwired: 1 in, 1 out]
                n473 = for {
                  tunnel: w991 -> [w997]
                  tunnel: w990 -> [w998] mode=indexing
                  tunnel: [w996] -> w984 mode=indexing
                  n474 = Index Array(array=w997, index=w998) -> (element=w996:string)
                }
                n475 = Unbundle By Name(w988) -> ("WP_ID"=w973:i32, "PS_ID"=w972:i32)
                n476 = Format Date/Time String(time format string (%c)=w978, seconds (now)="Results.TimeTo") -> (date/time string=w977:string)  [unwired: 1 in]
                n477 = Format Date/Time String(time format string (%c)=w978, seconds (now)="Results.TimeFrom") -> (date/time string=w976:string)  [unwired: 1 in]
                n478 = call "ProdaNG.Products.Get.vi"("Time To"=w977, "Time From"=w976, "error in (no error)"=w989, "proccessStepId (0: all)"=w972, "wabcoPartId"=w973, "dbHandleIn"=w981) -> ("error out"=w986:errorcluster, "Serials"=w974:string[], "Products"=w971:T1[], "dbHandle"=w987:i32)  [unwired: 2 in]
                "Products" <- w971
                n479 = Array Size(array=w971) -> (size(s)=w970:i32)
                n480 = Format Into String(format string="Products #%d" ("Caption.Text"), w970) -> (resulting string=w968:string)  [unwired: 2 in, 1 out]
                n481 = for {
                  tunnel: w974 -> [w995]
                  tunnel: w984 -> [w994] mode=indexing
                  tunnel: [w993] -> w983 mode=indexing if=w992
                  n482 = Search 1D Array(1D array=w995, element=w994) -> (index of element=w993:i32)  [unwired: 1 in]
                  n483 = Greater Or Equal To 0?(x=w993) -> (x >= 0?=w992:bool)
                }
                n484 = property on="ProductList" class="LstBox (strict)"("Caption.Text"=w968) -> ()  [unwired: 2 in, 2 out]
                n485 = property on="ProductList" class="LstBox (strict)"(error in=w986, "Item Names"=w974, "Val(Sgnl)"=w983, "Top Row"=0) -> (error out=w985:errorcluster)  [unwired: 1 in, 1 out]
              }
              frame #4 {
                w999 = FALSE ("Value (Signaling)")
                n486 = property on="ResultsTree" class="Tree (strict)"(error in=w1003, "Val(Sgnl)"=w1005, "TopLeft"=w1004) -> (error out=w1002:errorcluster)  [unwired: 1 in, 1 out]
                n487 = property on="ButtonRefreshResultTree" class="Bool (strict)"("Value"=w999) -> ()  [unwired: 2 in, 2 out]
                n488 = local read "FPref"() -> (w1000:refnum<vi>)
                n489 = property class="Pnl"(reference=w1000, "DeferPanUpdts"=FALSE ("Defer Panel Updates")) -> ()  [unwired: 1 in, 2 out]
                n490 = property on="Progress" class="Bool (strict)"("Visible"=w999) -> ()  [unwired: 2 in, 2 out]
                n491 = property on="Hider" class="Bool (strict)"("Visible"=w999) -> ()  [unwired: 2 in, 2 out]
              }
            }
          }
          event "ResultsAmount": Value Change {
            n492 = event-data() -> ()  [unwired: 1 in, 1 out]
            n493 = property on="ResultsSpan" class="Enum (strict)"() -> ("Value"=w1015:T15)  [unwired: 2 in, 2 out]
            n494 = Equal?(x=w1015, y=T15."Custom") -> (x = y?=w1006:bool)
            n495 = property on="ButtonRefreshResultTree" class="Bool (strict)"("Val(Sgnl)"=TRUE ("Value (Signaling)")) -> ()  [unwired: 2 in, 2 out]
            n496 = Select(t=T11."Disabled and Grayed Out" ("Disabled"), s=w1006, f=T11."Enabled" ("Disabled")) -> (s? t:f=w1011:T11)
            n497 = Select(t=T11."Enabled" ("Disabled"), s=w1006, f=T11."Disabled and Grayed Out" ("Disabled")) -> (s? t:f=w1008:T11)
            n498 = property on="ResultsAmount" class="DigNum (strict)"("DisabledEnum"=w1011) -> ()  [unwired: 2 in, 2 out]
            n499 = property on="Results.TimeFrom" class="AbsTime (strict)"("DisabledEnum"=w1008) -> (error out=w1007:errorcluster)  [unwired: 2 in, 1 out]
            n500 = case shown="True" w1006 {
              frame False {
              }
              frame True {
                n501 = invoke on="Results.TimeTo" class="AbsTime (strict)" method="Reinit To Default"() -> (error out=w1020:errorcluster)  [unwired: 3 in, 2 out]
                n502 = invoke on="Results.TimeFrom" class="AbsTime (strict)" method="Reinit To Default"(error in=w1020) -> ()  [unwired: 2 in, 3 out]
              }
            }
            n503 = property on="Results.TimeTo" class="AbsTime (strict)"(error in=w1007, "DisabledEnum"=w1008) -> ()  [unwired: 1 in, 2 out]
          }
          event "Results.TimeFrom", "Results.TimeTo": Value Change {
            w1021 = T11."Enabled" ("Disabled")
            n504 = event-data() -> ()  [unwired: 1 in, 1 out]
            n505 = property on="ButtonRefreshResultTree" class="Bool (strict)"("Val(Sgnl)"=TRUE ("Value (Signaling)")) -> ()  [unwired: 2 in, 2 out]
            n506 = property on="ResultsSpan" class="Enum (strict)"("Value"=ProdaNG.Configurator.ResultsTimeSpan."Custom" ("ResultsSpan")) -> ()  [unwired: 2 in, 2 out]
            n507 = property on="ResultsAmount" class="DigNum (strict)"("DisabledEnum"=T11."Disabled and Grayed Out" ("Disabled")) -> ()  [unwired: 2 in, 2 out]
            n508 = property on="Results.TimeFrom" class="AbsTime (strict)"("DisabledEnum"=w1021) -> (error out=w1022:errorcluster)  [unwired: 2 in, 1 out]
            n509 = property on="Results.TimeTo" class="AbsTime (strict)"(error in=w1022, "DisabledEnum"=w1021) -> ()  [unwired: 1 in, 2 out]
          }
          event "ProductListSelectAll": Value Change {
            n510 = event-data() -> ()  [unwired: 1 in, 1 out]
            n511 = case shown="\"True\"" "ProductListSelectAll" {
              tunnel: [i32[] [] ("Value (Signaling)") w1037] -> w1032
              tunnel: [enum8{"False", "True", "Mixed"}."False" ("ProductListSelectAll") enum8{"False", "True", "Mixed"}."True" ("ProductListSelectAll")] -> w1031
              frame "False", "Mixed" {
              }
              frame "True" {
                n512 = property on="ProductList" class="LstBox (strict)"() -> ("Item Names"=w1038:string[])  [unwired: 2 in, 2 out]
                n513 = for {
                  tunnel: w1038 -> [_] mode=indexing
                  tunnel: [w1040] -> w1037 mode=indexing
                  i -> [w1040]
                }
              }
            }
            n514 = property on="ProductListSelectAll" class="MixedCheckbox (strict)"("Value"=w1031) -> ()  [unwired: 2 in, 2 out]
            n515 = property on="ProductList" class="LstBox (strict)"("Val(Sgnl)"=w1032) -> ()  [unwired: 2 in, 2 out]
          }
          event "ProductList": Value Change {
            n516 = event-data() -> ()  [unwired: 1 in, 1 out]
            n517 = stacked-sequence {
              tunnel: [_ _ _ _ w1079 _] -> w1042
              tunnel: w1043 -> [_ _ _ _ w1078 _]
              tunnel: w1044 -> [_ _ _ _ w1084 _]
              tunnel: [_ _ _ _ w1080 _] -> w1041
              tunnel: [_ _ _ w1060 _ _] -> _
              frame #0 {
                w1046 = TRUE ("Value (Signaling)")
                n518 = property on="ButtonRefreshResultTree" class="Bool (strict)"("Value"=w1046) -> ()  [unwired: 2 in, 2 out]
                n519 = property on="Progress" class="Bool (strict)"("Visible"=w1046) -> ()  [unwired: 2 in, 2 out]
                n520 = property on="Hider" class="Bool (strict)"("Visible"=w1046) -> ()  [unwired: 2 in, 2 out]
              }
              frame #1 {
                n521 = local read "FPref"() -> (w1047:refnum<vi>)
                n522 = property class="Pnl"(reference=w1047, "DeferPanUpdts"=TRUE ("Defer Panel Updates")) -> ()  [unwired: 1 in, 2 out]
              }
              frame #2 {
                n523 = property on="ProductList" class="LstBox (strict)"() -> ("Item Names"=w1058:string[])  [unwired: 2 in, 2 out]
                n524 = Array Size(array=w1058) -> (size(s)=w1057:i32)
                n525 = Array Size(array="ProductList") -> (size(s)=w1056:i32)
                n526 = Equal?(x=w1056, y=w1057) -> (x = y?=w1054:bool)
                n527 = Less Or Equal To 0?(x=w1056) -> (x <= 0?=w1050:bool)
                n528 = Select(t=enum8{"False", "True", "Mixed"}."True" ("Mixed Checkbox"), s=w1054, f=enum8{"False", "True", "Mixed"}."Mixed" ("Mixed Checkbox")) -> (s? t:f=w1051:enum8{"False", "True", "Mixed"})
                n529 = Select(t=enum8{"False", "True", "Mixed"}."False" ("Mixed Checkbox"), s=w1050, f=w1051) -> (s? t:f=w1049:enum8{"False", "True", "Mixed"})
                n530 = property on="ProductListSelectAll" class="MixedCheckbox (strict)"("Value"=w1049) -> ()  [unwired: 2 in, 2 out]
              }
              frame #3 {
                w1062 = -2 ("Active Item:Row Number")
                n531 = invoke on="ResultsTree" class="Tree (strict)" method="Edit Tree Items.Delete"("tag"="", "Delete Children"=TRUE ("Delete Children?")) -> (error out=w1064:errorcluster)  [unwired: 3 in, 4 out]
                n532 = property on="ResultsTree" class="Tree (strict)"(error in=w1064, "Active Item Row Number"=w1062, "ActiveColNum"=w1062, "CellBG"=u32 16448250) -> (error out=w1063:errorcluster)  [unwired: 1 in, 1 out]
                n533 = for {
                  N: 50 -> [_]
                  tunnel: string[] ["Name", "Order", "Low Limit", "High Limit"] -> [w1072]
                  shift-right: [w1070] -> w1060
                  shift-left: w1063 -> [w1075]
                  i -> [w1069]
                  n534 = Index Array(array=w1072, index=w1069) -> (element=w1071:string)
                  n535 = property on="ResultsTree" class="Tree (strict)"(error in=w1075, "Active Item Row Number"=-1 ("Active Item:Row Number"), "ActiveColNum"=w1069, "CellBG"=u32 13816530, "Cell String"=w1071) -> (error out=w1070:errorcluster)  [unwired: 1 in, 1 out]
                }
              }
              frame #4 {
                n536 = property on="ProductList" class="LstBox (strict)" props=["Item Names", "Value"](error in=w1084) -> (error out=w1081:errorcluster, "Value"=w1085:i32[])  [unwired: 1 in, 2 out]
                n537 = local read "Products"() -> (w1077:T1[])
                n538 = for {
                  tunnel: w1077 -> [w1087]
                  tunnel: w1085 -> [w1088] mode=indexing
                  tunnel: [w1086] -> w1076 mode=indexing
                  n539 = Index Array(array=w1087, index=w1088) -> (element=w1086:T1)
                }
                n540 = local read "Identification"() -> (w1082:T7)
                n541 = control-ref of="ResultsTree"() -> (w1083:refnum<vi>)
                n542 = call "ProdaNG.Tree.Results.Update.vi"("Identification"=w1082, "Products"=w1076, "TreeControl in"=w1083, "error in (no error)"=w1081, "dbHandle in"=w1078) -> ("error out"=w1080:errorcluster, "dbHandle out"=w1079:i32)  [unwired: 4 in, 1 out]
              }
              frame #5 {
                w1089 = FALSE ("Value (Signaling)")
                n543 = property on="ButtonRefreshResultTree" class="Bool (strict)"("Value"=w1089) -> ()  [unwired: 2 in, 2 out]
                n544 = local read "FPref"() -> (w1090:refnum<vi>)
                n545 = property class="Pnl"(reference=w1090, "DeferPanUpdts"=FALSE ("Defer Panel Updates")) -> ()  [unwired: 1 in, 2 out]
                n546 = property on="Progress" class="Bool (strict)"("Visible"=w1089) -> ()  [unwired: 2 in, 2 out]
                n547 = property on="Hider" class="Bool (strict)"("Visible"=w1089) -> ()  [unwired: 2 in, 2 out]
              }
            }
          }
        }
        n548 = call <vilib>:"General Error Handler Core CORE.vi"("type of dialog (OK msg:1)"=DialogTypeEnum."continue or stop message", "error in (no error)"=w71) -> ("stop event propagated"=w67:bool, "error out"=w70:errorcluster)  [unwired: 12 in, 4 out]
        n549 = Compound Arithmetic op=OR(w67, w69) -> (w68:bool)
        n550 = call <vilib>:"Clear Errors.vi"("error in (no error)"=w70) -> ("error out"=w72:errorcluster)  [unwired: 5 in, 1 out]
      }
      n551 = call "ProdaNG.LogOut.vi"("error in"=w63, "dbHandleIn"=w64) -> ("error out"=w61:errorcluster)  [unwired: 9 in]
      n552 = call "ProdaNG.Exit.vi"("error in (no error)"=w61) -> ("error out"=w60:errorcluster)  [unwired: 10 in]
    }
    frame #2 {
      w1092 = TRUE ("Value (Signaling)")
      w1096 = -2 ("Active Item:Row Number")
      w1110 = T11."Enabled" ("Disabled")
      w1109 = FALSE ("ButtonPartList")
      w1105 = ""
      w1113 = TRUE ("Delete Children?")
      w1114 = ""
      w1103 = FALSE ("Visible")
      n553 = control-ref of="TestTree"() -> (w1117:refnum<vi>)
      n554 = invoke on="TestTree" class="Tree (strict)" method="Edit Tree Items.Delete"("tag"=w1114, "Delete Children"=w1113) -> (error out=w1116:errorcluster)  [unwired: 3 in, 4 out]
      n555 = call "ProdaNG.Tree.Clear.vi"("TestStepsTree"=w1117) -> ()  [unwired: 10 in, 1 out]
      n556 = property on="ProductList" class="LstBox (strict)"("Item Names"=string[] [], "Value"=i32[] [] ("ProductList"), "Top Row"=0) -> ()  [unwired: 2 in, 2 out]
      n557 = property on="FileInUse" class="Str"("Caption.Text"="", "Text.BGColor"=u32 13816530) -> ()  [unwired: 2 in, 2 out]
      n558 = invoke on="ProcTree" class="Tree (strict)" method="Edit Tree Items.Delete"(error in=w1116, "tag"=w1114, "Delete Children"=w1113) -> (error out=w1115:errorcluster)  [unwired: 2 in, 4 out]
      n559 = local write "MainTab"(enum32{"Parts", "Test", "Results"}."Parts" ("MainTab")) -> ()
      n560 = property on="MainTab" class="TabCtl (strict)"("Page Labels Display Visible?"=TRUE) -> ()  [unwired: 2 in, 2 out]
      n561 = local write "DBStatus"(w1105) -> ()
      n562 = local write "Identification"(T12 {"processId"=0, "systemId"=0, "processStepId"=0, "wabcoPartId"=0} ("Identification")) -> ()
      n563 = property on="ButtonRefreshResultTree" class="Bool (strict)"("Value"=w1092) -> ()  [unwired: 2 in, 2 out]
      n564 = invoke on="ResultsTree" class="Tree (strict)" method="Edit Tree Items.Delete"(error in=w1115, "tag"=w1114, "Delete Children"=w1113) -> (error out=w1094:errorcluster)  [unwired: 2 in, 4 out]
      n565 = property on="ButtonParts" class="Bool (strict)"("Value"=w1109) -> (error out=w1108:errorcluster)  [unwired: 2 in, 1 out]
      n566 = local write "Status"(w1105) -> ()
      n567 = local read "FPref"() -> (w1119:refnum<vi>)
      n568 = property on="Progress" class="Bool (strict)"("Visible"=w1103) -> ()  [unwired: 2 in, 2 out]
      n569 = property on="ButtonTest" class="Bool (strict)"(error in=w1108, "Value"=w1109, "DisabledEnum"=w1110) -> (error out=w1107:errorcluster)  [unwired: 1 in, 1 out]
      n570 = property on="ButtonRefreshTestTree" class="Bool (strict)"("Value"=w1092) -> ()  [unwired: 2 in, 2 out]
      n571 = property on="Hider" class="Bool (strict)"("Visible"=w1103) -> ()  [unwired: 2 in, 2 out]
      n572 = Close Reference(reference=w1119) -> ()  [unwired: 1 in, 1 out]
      n573 = property on="ButtonResults" class="Bool (strict)"(error in=w1107, "Value"=w1109, "DisabledEnum"=w1110) -> ()  [unwired: 1 in, 2 out]
      n574 = property on="HiderParts" class="Bool (strict)"("Visible"=w1103) -> ()  [unwired: 2 in, 2 out]
      n575 = property on="ResultsTree" class="Tree (strict)"(error in=w1094, "Active Item Row Number"=w1096, "ActiveColNum"=w1096, "CellBG"=u32 16448250) -> (error out=w1097:errorcluster)  [unwired: 1 in, 1 out]
      n576 = property on="ButtonRefreshTreeProc" class="Bool (strict)"("Value"=w1092) -> ()  [unwired: 2 in, 2 out]
      n577 = property on="ButtonConnect" class="Bool (strict)"("Value"=w1103) -> ()  [unwired: 2 in, 2 out]
      n578 = property on="ProductListSelectAll" class="MixedCheckbox (strict)"("Value"=enum8{"False", "True", "Mixed"}."False" ("Mixed Checkbox")) -> ()  [unwired: 2 in, 2 out]
      n579 = for {
        N: 50 -> [_]
        tunnel: string[] ["Name", "Order", "Low Limit", "High Limit"] -> [w1123]
        shift-right: [w1121] -> _
        shift-left: w1097 -> [w1126]
        i -> [w1120]
        n580 = Index Array(array=w1123, index=w1120) -> (element=w1122:string)
        n581 = property on="ResultsTree" class="Tree (strict)"(error in=w1126, "Active Item Row Number"=-1 ("Active Item:Row Number"), "ActiveColNum"=w1120, "CellBG"=u32 13816530, "Cell String"=w1122) -> (error out=w1121:errorcluster)  [unwired: 1 in, 1 out]
      }
      n582 = property on="Process Found" class="Bool (strict)"("Value"=w1103) -> ()  [unwired: 2 in, 2 out]
    }
  }
